vi "Text control 2 v3.2.vi"() -> ()   [LabVIEW 2016]
panel:
  out "I vs Vd":cluster{"Y data in":dbl[], "X data in":dbl[]}[](graph)
  in  "Auto Reset":bool
  in  "Reset":bool
  out "Id min vs time":cluster{"Y data in":dbl[], "X data in":dbl[]}[](graph)
  in  "Time Offset":dbl caption="Set Start Time (s)"
  out "Total lines":i32
  out "Line running":i32
  in  "byte count":u32=64
  in  "Serial End Mode for Reads":u16(ring)=2 items=["None", "LastBit", "TermChar"]
  in  "Timeout (ms)":u32=10000
  in  "Enable Termination\nChar (T)":bool=TRUE
  in  "Termination char\n(0xA = '\\n' = LF)\n(0xD = '\\r' = CR)":u8=13 format="%.0x"
  in  "flow control":u16(ring) items=["None"=0, "XON/XOFF"=1, "RTS/CTS"=2, "DTR/DSR"=4]
  in  "stop bits":u16(ring)=10 items=["1.0"=10, "1.5"=15, "2.0"=20]
  in  "parity":u16(ring) items=["None", "Odd", "Even", "Mark", "Space"]
  in  "data bits":u16=8 min=5 max=8 step=1
  in  "VISA resource name":refnum<visa-resource-name>="COM6"
  in  "baud rate":u32=9600
  out "Serial port output":string
  out "error out":errorcluster
  in  "Units":u16(ring) items=["Seconds", "Minutes", "Hours"]
  out "Elapsed Time":dbl caption="Elapsed Time (s)"
  out "Id max vs time":cluster{"Y data in":dbl[], "X data in":dbl[]}[](graph)
  out "Ig":dbl format="%.2e"
  out "Id":dbl format="%.2e"
  out "Is":dbl format="%.2e"
  out "I vs Vg":cluster{"Y data in":dbl[], "X data in":dbl[]}[](graph)
  in  "Panel Controls 2":T1={"Emergency Stop"=refnum, "TransGraph Max"=1e-05, "Text/Graph (text=false)"=TRUE, "TransGraph Min"=1e-11} {"TransGraph Min" format="%.2e"; "TransGraph Max" format="%.2e"}
  out "Command running:":string="#output s 0 0 0 -0.008 0.008 0.002"
  in  "Standby":T2
  in  "Full Reset":bool
  in  "SMU4":cluster{"on/off":bool, "Voltage":dbl} {"Voltage" min=-100.0 max=100.0 format="%.2f"}
  in  "Source/Drain Range":u8(slide)=6 max=11 scale=0.0..11.0
  in  "Source/Drain\nRange mode":u16(ring) items=["Auto", "Limited", "Fixed"]
  in  "Gate Range":u8(slide)=6 max=11 scale=0.0..11.0
  in  "Gate Range\nmode":u16(ring) items=["Auto", "Limited", "Fixed"]
  in  "Gate":T3={"Gate Start"=0.0, "Gate Stop"=2.0, "Gate Step (linear only)"=1.0, "Gate Compliance"=0.0001, "Gate PComp"=0.0, "Range mode"=0, "Range"=6} {"Range" max=11 scale=0.0..11.0; "Range mode" items=["Auto", "Limited", "Fixed"]; "Gate PComp" format="%^.2e"; "Gate Compliance" format="%^.2e"; "Gate Step (linear only)" format="%^.4e"; "Gate Stop" format="%^.4e"; "Gate Start" format="%^.4e"}
  in  "Drain 2":T4={"Drain Start"=0.0, "Drain Stop"=2.0, "Drain Compliance"=0.0001, "Drain Step"=1.0, "Drain PComp"=0.0, "Range mode"=0, "Range"=6} {"Range" max=11 scale=0.0..11.0; "Range mode" items=["Auto", "Limited", "Fixed"]; "Drain PComp" format="%^.2e"; "Drain Step" format="%^.4e"; "Drain Compliance" format="%^.2e"; "Drain Stop" format="%^.4e"; "Drain Start" format="%^.4e"}
  in  "Timings 2":T5={"integration time"=0, "Short/Long integration time"=0.00064, "hold time (sec)"=0.0, "delay time (sec)"=0.0, "Step Time (0 disables)"=0.0, "sweep method"=0, "Pulse period"=0.005, "Base voltage"=0.0, "Pulse width"=0.0005} {"Pulse width" min=0.0005 max=0.1 step=0.0001 format="%.4f"; "Base voltage" format="%^.4e"; "Pulse period" min=0.005 max=1.0 step=0.0001 format="%.4f"; "sweep method" items=["Continuous", "Pulsed"]; "Step Time (0 disables)" format="%.2f"; "delay time (sec)" format="%.4f"; "hold time (sec)" format="%.4f"; "Short/Long integration time" format="%^.0e"; "integration time" scale=0.0..2.0}
  in  "Panel Controls":T6={"Emergency Stop"=refnum, "TransGraph Max"=1e-05, "Text/Graph (text=false)"=TRUE} {"TransGraph Max" format="%.2e"}
  in  "Interrupt run":bool
  in  "Drain: Compliance":dbl=0.001 format="%.8f"
  in  "Gate: Compliance":dbl=0.001 format="%.8f"
  out "Path":path=path "C:/users/rlp38/09Apr2009LTtesting/test2.txt"
  in  "hold time /s":dbl format="%.2f"
  in  "delay time /s":dbl format="%.2f"
  in  "integration time":u32(slide) max=2 step=1 scale=0.0..2.0
  in  "Integration time (short)":dbl=0.0019 min=8e-05 max=0.0019 step=8e-05 format="%^.0e"
  in  "Integration time (long)":dbl=0.32 min=0.04 max=2.0 step=0.02 format="%.2f"
  in  "Step delay /s":dbl format="%.2f"
  in  "Program":string="#pulsedstressV d 0.03 20 0 0.5 0.0827 5\n#\n#itime s\n#gaterangemode l\n#drainrangemode l\n#pulsed on 0.05 0 0.02\n#transfer d 1 -1 -0.1 -1 -1 0\n#wait-min 1\n#transfer d 1 -1 -0.1 -1 -1 0\n#output d 0 -1 -0.5 0 -1 -0.1\n#transfer d -10 40 1 5 40 35\n#transfer d -10 40 1 5 40 35\n#output d 0 40 20 0 40 1\n#\n#\n#sample 1 0.008 221 6 0.003\n#samplei 400e-6 200 6 0.002 0.1\n#vsu2pulse -10 4\n#\n#stressV 0.016 0.03 2e-4 0.1e-3 11\n#stressI 220e-7 0.08 15\n#transfer s -1 1 0.5 -0.005 0.005 0.005\n#output s 0 0 0 -0.008 0.008 0.002\n"
  # "Serial port settings"
  # "Time"
  # "100 samples is approx 13s with medium integration"
  # "Syntax:\nitime [s|m|l]\ngaterangemode [a|l|f]\ndrainrangemode [a|l|f]\npulsed [on|off] PulsePeriod(sec) PulseBaseVoltage PulseONWidth(sec)\nstandby [on l off]\nwait NumMilliseconds\nwait-min NumMinutes\n# texthere = comment\ntransfer [s|d] VgStart VgStop VgStep VdStart VdStop VdStep\noutput [s|d] VgStart VgStop VgStep VdStart VdStop VdStep\nsample Vg Vd NumSamples Time(s) SampleInterval(s)\nsamplei Idg NumSamples Time(s) SampleInterval(s) VDGcompliance\n# if in doubt use SampleInterval(s) = 0.004\nstressV VG VD IGcompliance IDcompliance Duration(sec)\nstressI IDG VDGcompliance Duration(sec)\nvsu2pulse Bias Duration(s)\npulsedstressV [s|d] VEstop VgON VgOFF Period(s) PulseONwidth(s) Vd\nsample-fpp Vg Vd NumSamples Time\nresample-fpp Vg Vd\ntransfer-fpp [s|d] VgStart VgStop VgStep VdStart VdStop VdStep\noutput-fpp [s|d] VgStart VgStop VgStep VdStart VdStop VdStep\nserial SerialPortCommand"
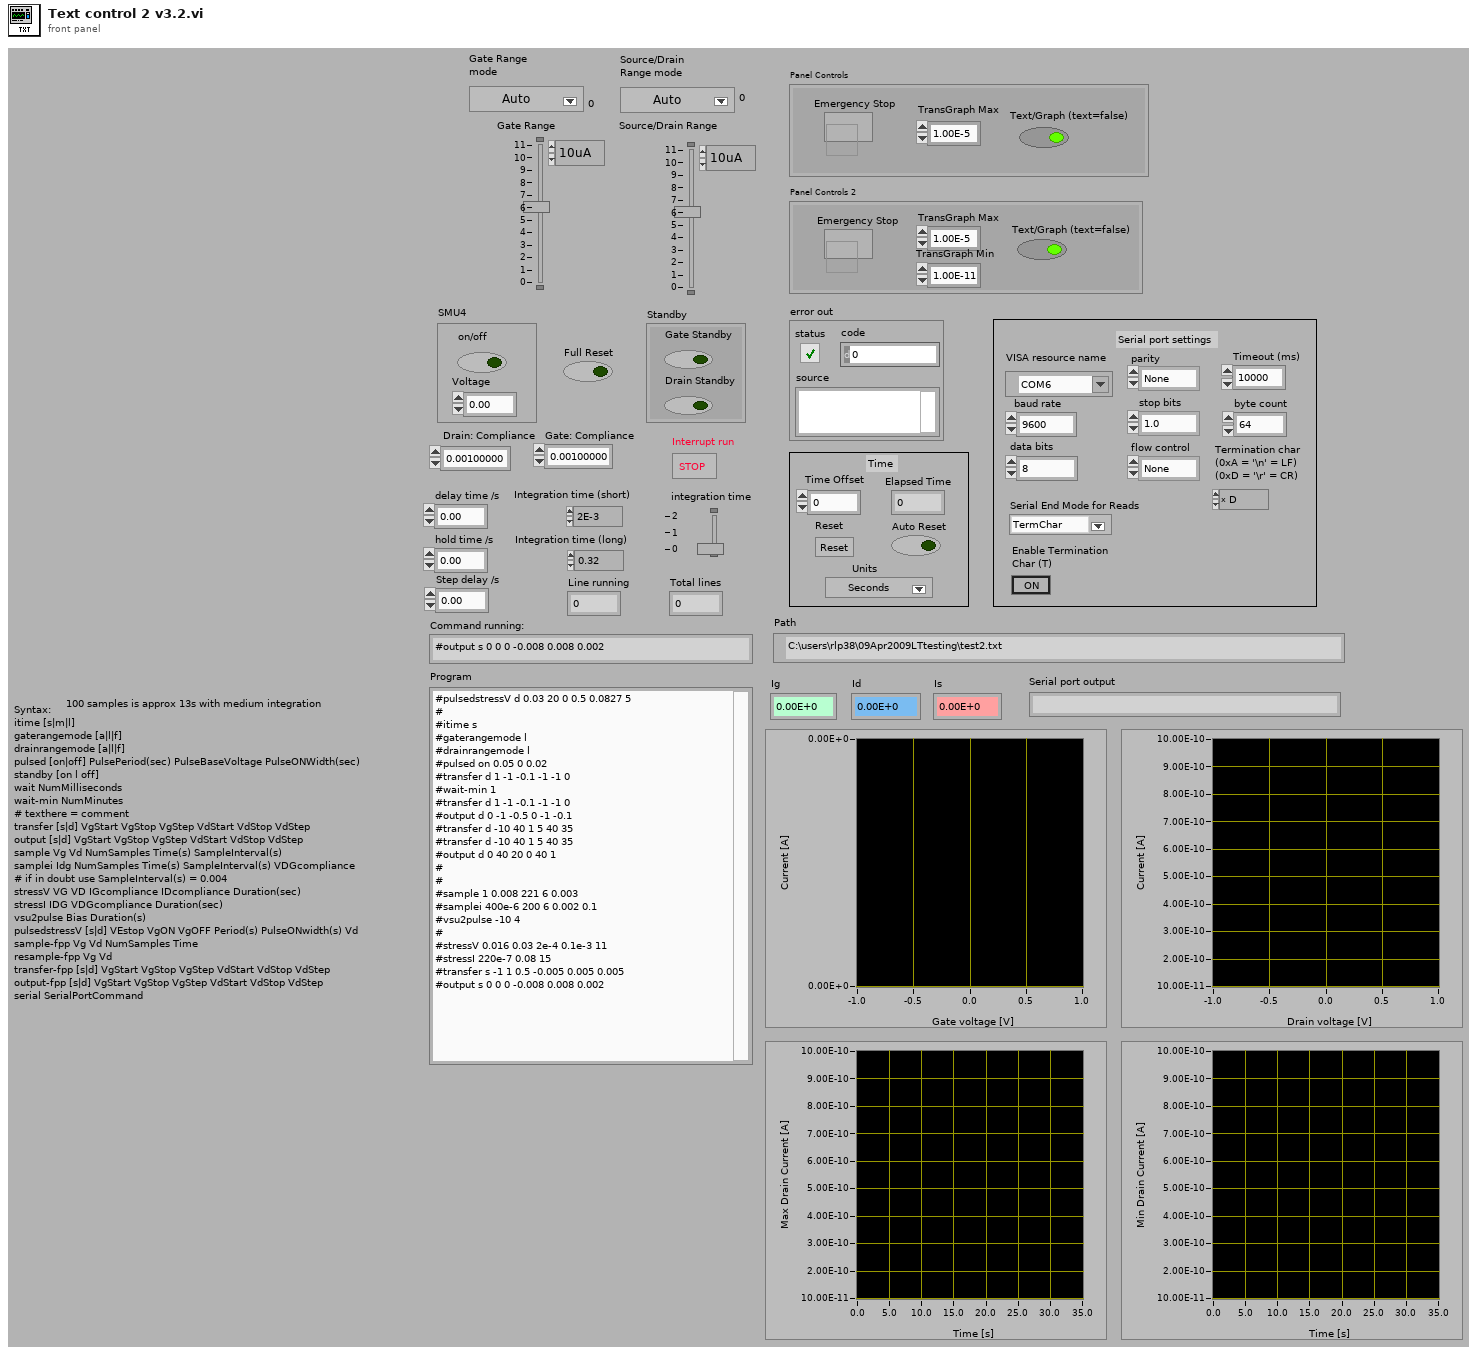
[diagram p1: front panel]
types:
  T1 = cluster{"Emergency Stop":refnum<vi>, "TransGraph Max":dbl, "Text/Graph (text=false)":bool, "TransGraph Min":dbl}
  T2 = cluster{"Gate Standby":bool, "Drain Standby":bool}
  T3 = cluster{"Gate Start":dbl, "Gate Stop":dbl, "Gate Step (linear only)":dbl, "Gate Compliance":dbl, "Gate PComp":dbl, "Range mode":u16, "Range":u8}
  T4 = cluster{"Drain Start":dbl, "Drain Stop":dbl, "Drain Compliance":dbl, "Drain Step":dbl, "Drain PComp":dbl, "Range mode":u16, "Range":u8}
  T5 = cluster{"integration time":u32, "Short/Long integration time":dbl, "hold time (sec)":dbl, "delay time (sec)":dbl, "Step Time (0 disables)":dbl, "sweep method":u16, "Pulse period":dbl, "Base voltage":dbl, "Pulse width":dbl}
  T6 = cluster{"Emergency Stop":refnum<vi>, "TransGraph Max":dbl, "Text/Graph (text=false)":bool}
  T7 = enum16{"open", "replace", "create", "open or create", "replace or create", "replace or create with confirmation"}
  T8 = cluster{"V2 Start":dbl, "V2 Step":dbl, "Number of points":i32}
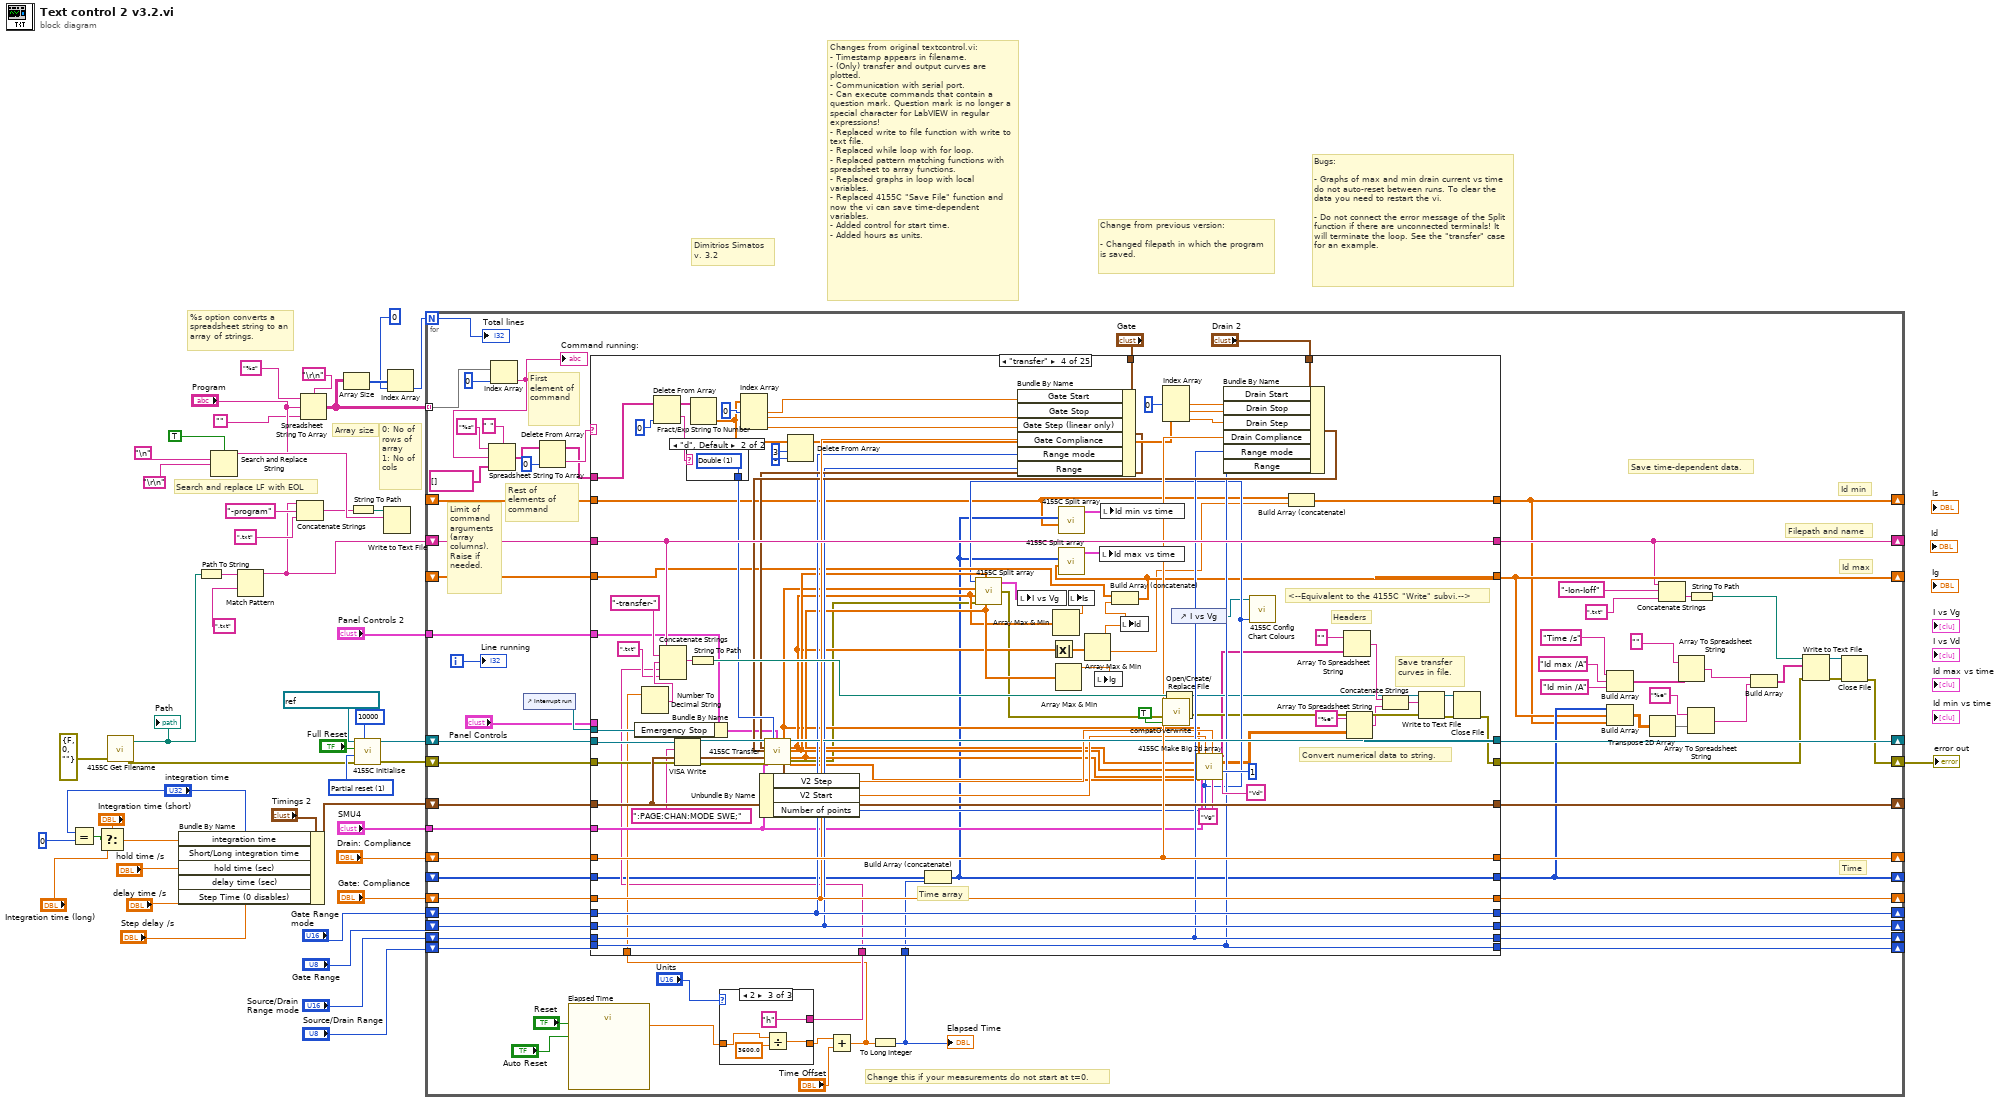
[diagram p0: block diagram]
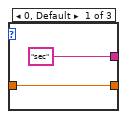
[diagram p2: hidden frame]
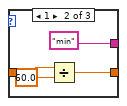
[diagram p3: hidden frame]
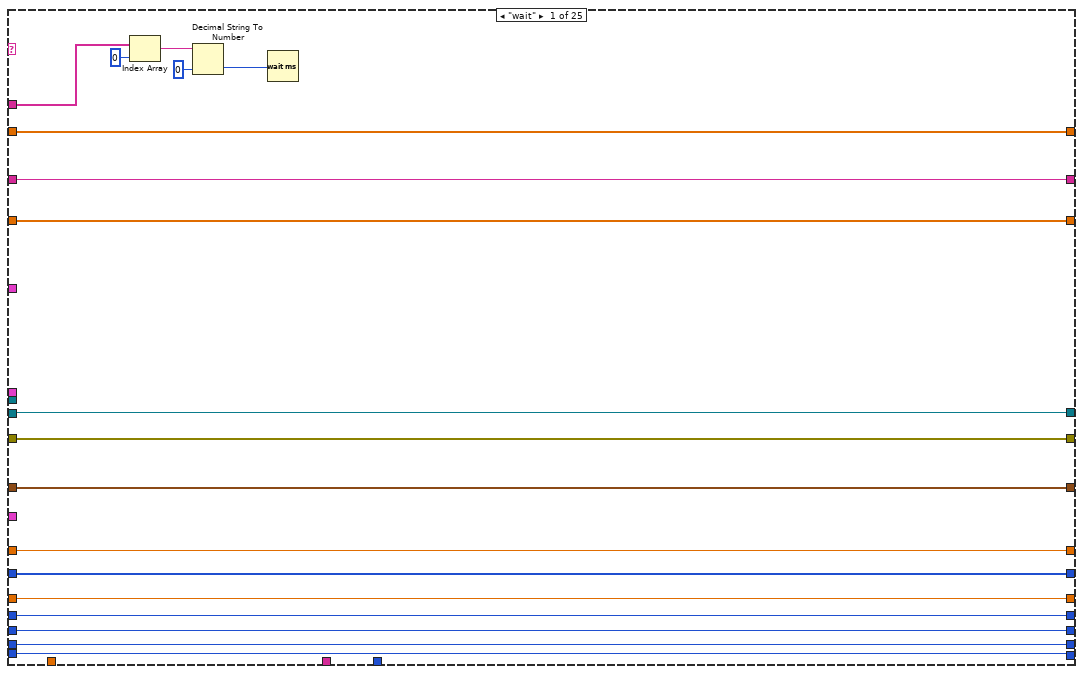
[diagram p4: hidden frame]
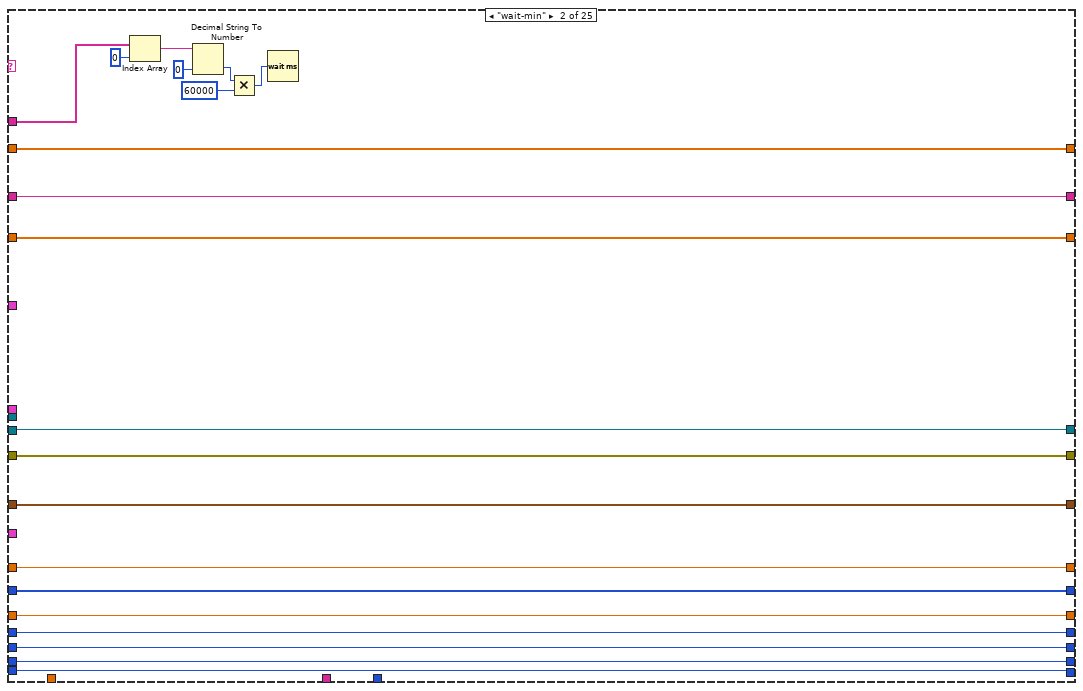
[diagram p5: hidden frame]
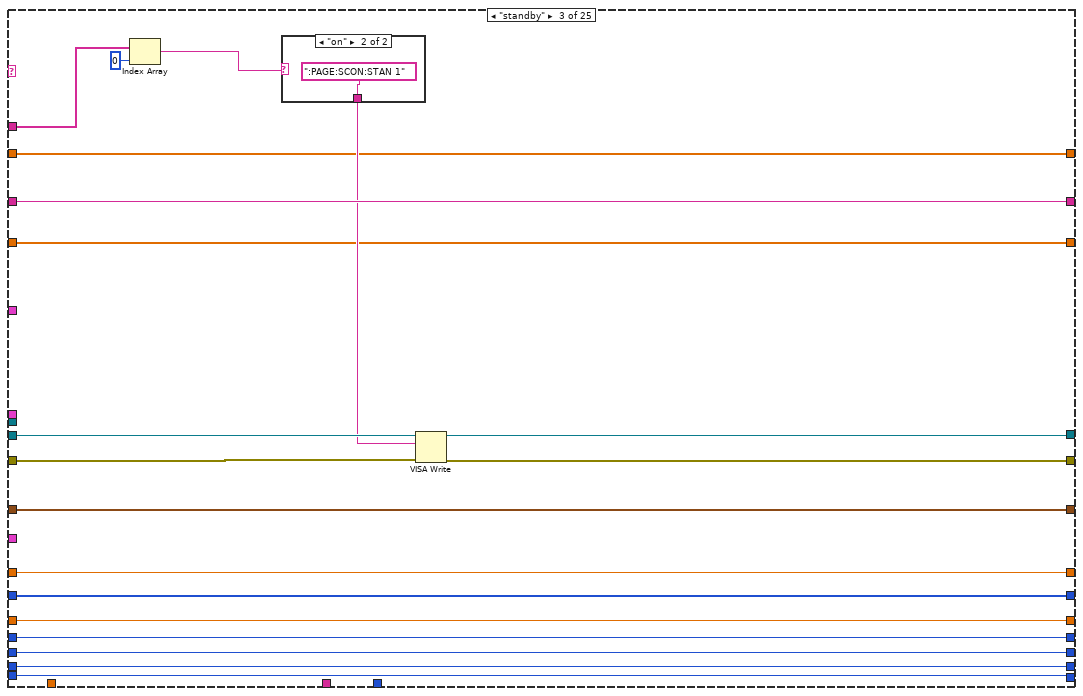
[diagram p6: hidden frame]
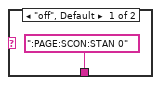
[diagram p7: hidden frame]
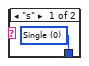
[diagram p8: hidden frame]
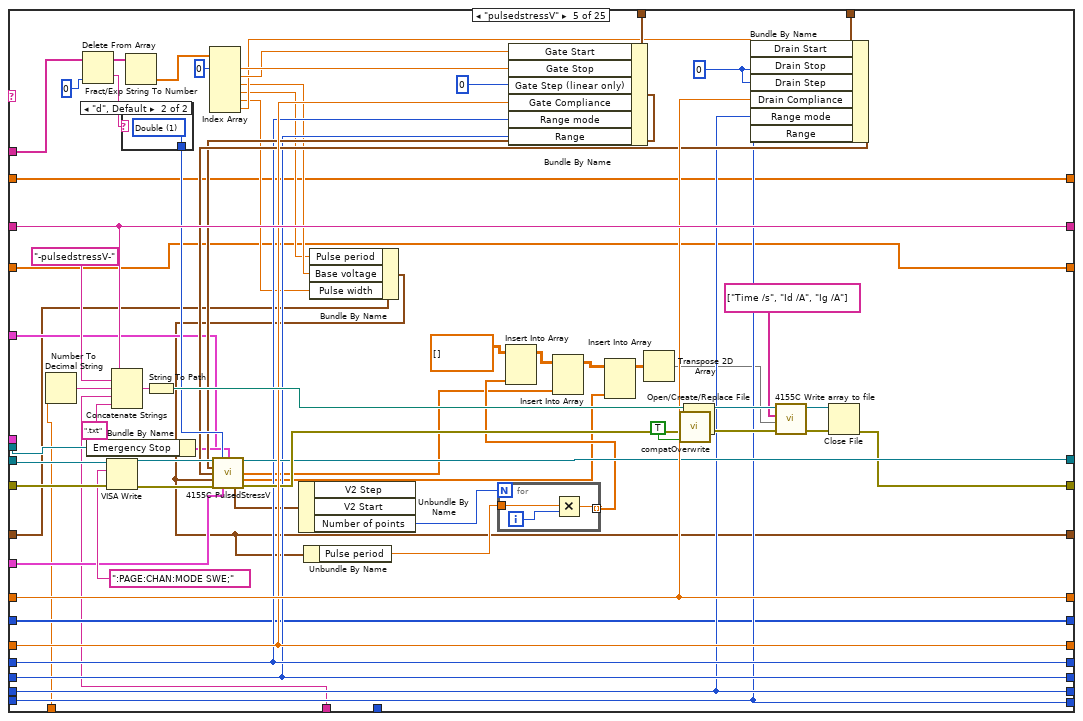
[diagram p9: hidden frame]
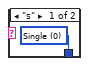
[diagram p10: hidden frame]
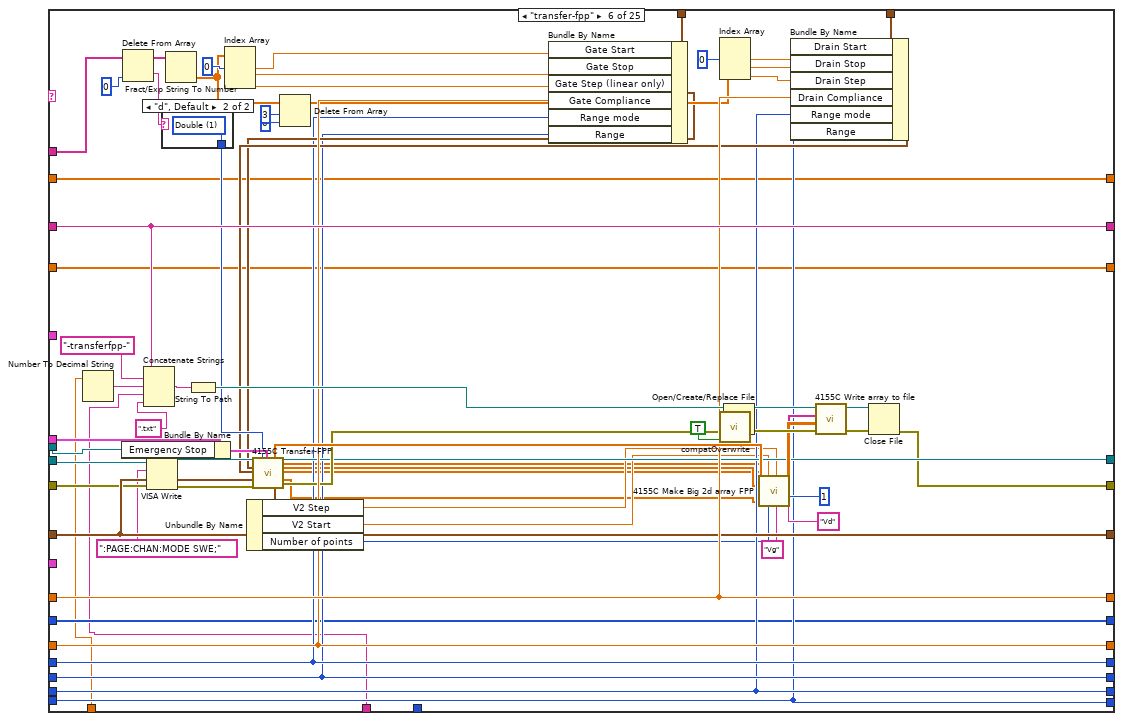
[diagram p11: hidden frame]
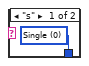
[diagram p12: hidden frame]
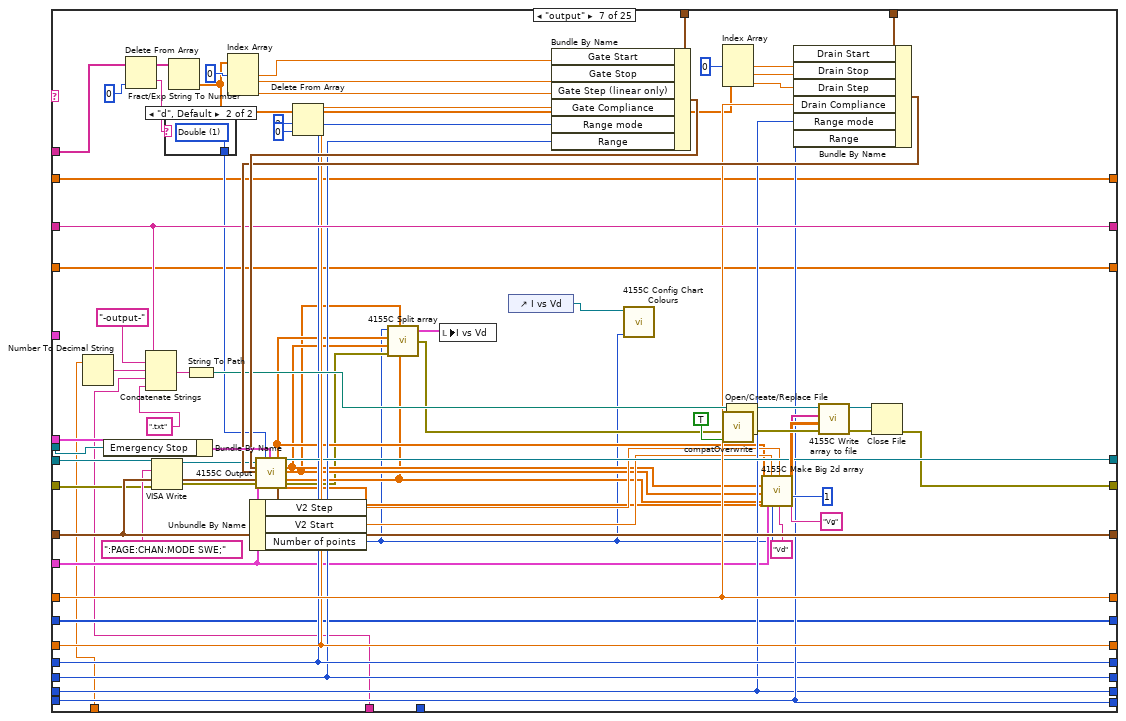
[diagram p13: hidden frame]
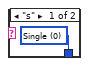
[diagram p14: hidden frame]
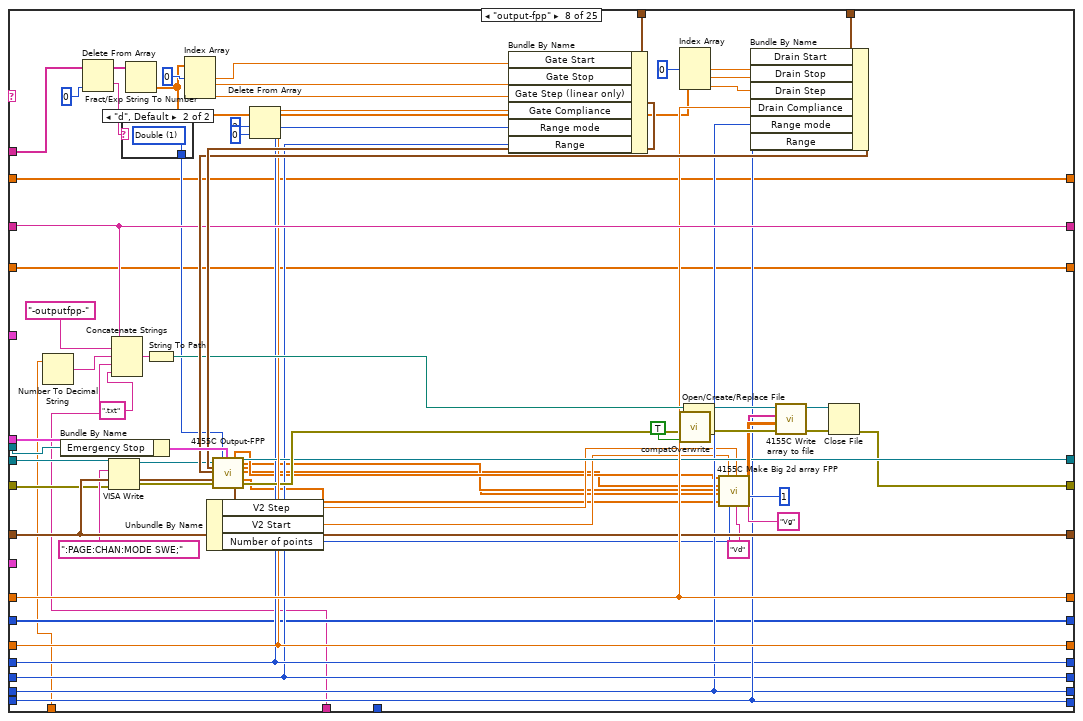
[diagram p15: hidden frame]
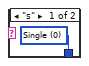
[diagram p16: hidden frame]
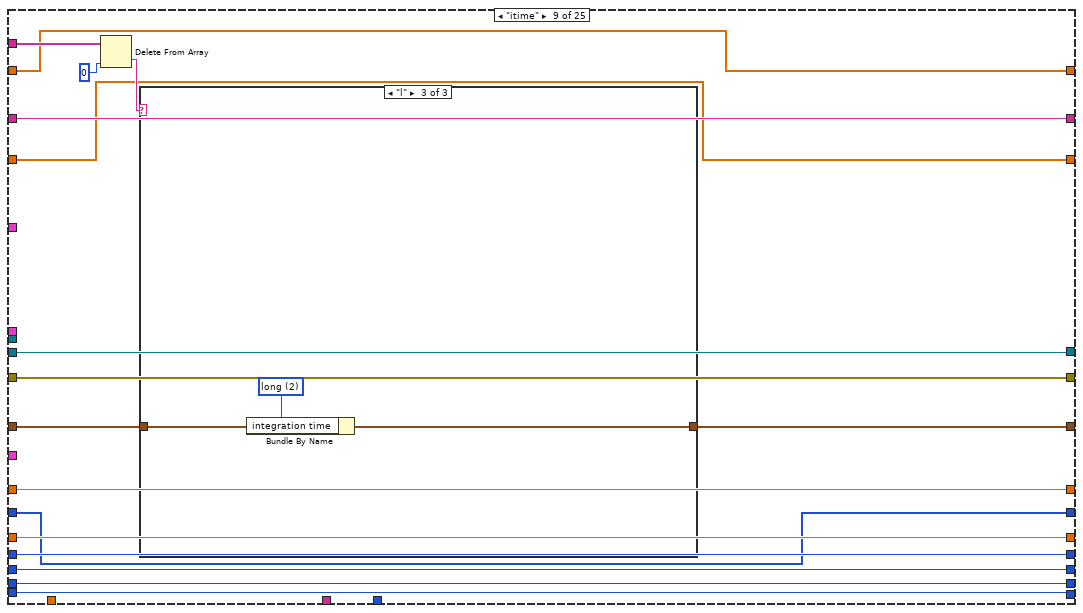
[diagram p17: hidden frame]
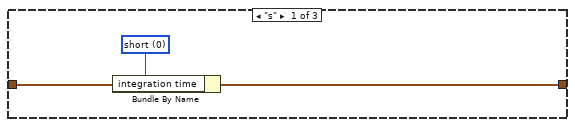
[diagram p18: hidden frame]
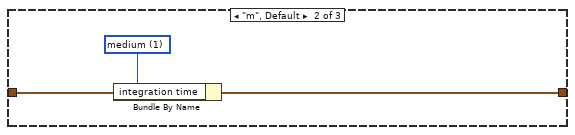
[diagram p19: hidden frame]
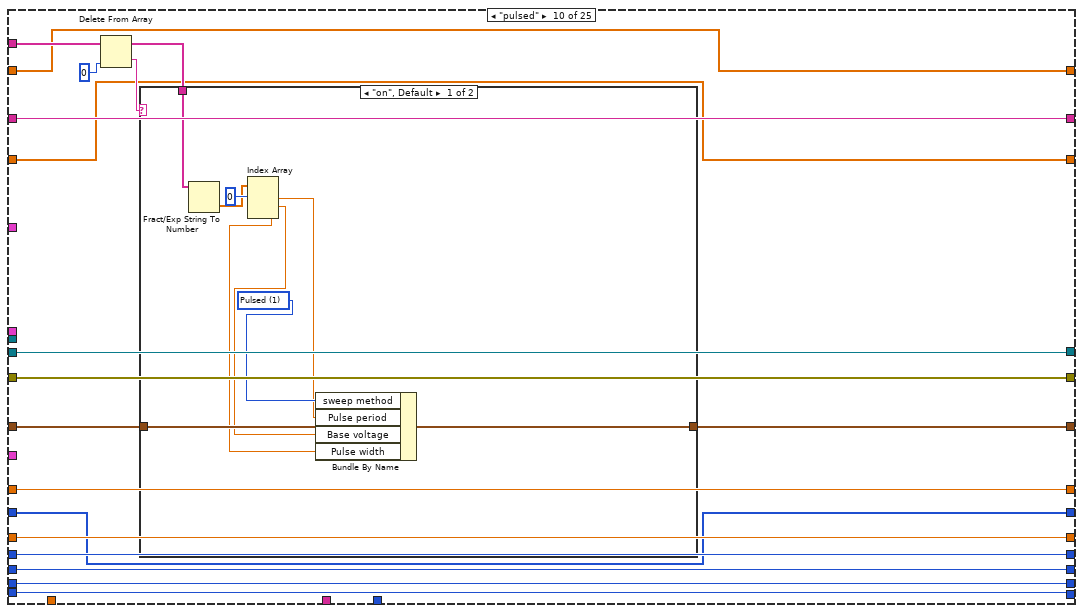
[diagram p20: hidden frame]
diagram:
  w39 = u16 1 items=["Reset All", "Partial reset"] ("Type of reset")
  # "Bugs:\n\n- Graphs of max and min drain current vs time do not auto-reset between runs. To clear the data you need to restart the vi.\n\n- Do not connect the error message of the Split function if there are unconnected terminals! It will terminate the loop. See the \"transfer\" case for an example."
  # "Array size"
  # "%s option converts a spreadsheet string to an array of strings."
  # "0: No of rows of array\n1: No of cols"
  # "Change from previous version:\n\n- Changed filepath in which the program is saved."
  # "Dimitrios Simatos\nv. 3.2"
  # "Changes from original textcontrol.vi:\n- Timestamp appears in filename.\n- (Only) transfer and output curves are plotted.\n- Communication with serial port.\n- Can execute commands that contain a question mark. Question mark is no longer a special character for LabVIEW in regular expressions!\n- Replaced write to file function with write to text file.\n- Replaced while loop with for loop.\n- Replaced pattern matching functions with spreadsheet to array functions.\n- Replaced graphs in loop with local variables.\n- Replaced 4155C \"Save File\" function and now the vi can save time-dependent variables.\n- Added control for start time.\n- Added hours as units."
  # "Search and replace LF with EOL"
  n1 = Equal?(x="integration time", y=u32 0) -> (x = y?=w43:bool)
  n2 = Select(t="Integration time (short)", s=w43, f="Integration time (long)") -> (s? t:f=w47:dbl)
  n3 = call "4155C Get Filename.vi"("error in (no error)"=errorcluster {"status"=FALSE, "code"=0, "source"=""}) -> ("error out"=w34:errorcluster, "path"=w8:path)  [unwired: 2 in, 1 out]
  "Path" <- w8
  n4 = Bundle By Name(cluster="Timings 2", "integration time"="integration time", "Short/Long integration time"=w47, "hold time (sec)"="hold time /s", "delay time (sec)"="delay time /s", "Step Time (0 disables)"="Step delay /s") -> (w31:T5)
  n5 = Path To String(path=w8) -> (string=w9:string)
  n6 = Search and Replace String(replace all?=TRUE ("replace all? (F)"), input string="Program", search string="\n", replace string="\r\n") -> (result string=w21:string)  [unwired: 4 in, 3 out]
  n7 = Match Pattern(string=w9, regular expression=".txt") -> (before substring=w3:string)  [unwired: 1 in, 3 out]
  n8 = Concatenate Strings(w3, "-program" ("Prefix"), ".txt" ("regular expression")) -> (w2:string)
  n9 = Spreadsheet String To Array(delimiter (Tab)="\r\n", format string="%s", spreadsheet string="Program", array type (2D Dbl)="") -> (array=w12:string[][])
  n10 = Array Size(array=w12) -> (size(s)=w16:i32[])
  n11 = String To Path(string=w2) -> (path=w1:path)
  n12 = call "4155C Initialise.vi"("VISA resource name in"=refnum<visa-resource-name> "GPIB0::14::INSTR", "Reset"="Full Reset", "Type of reset"=w39, "error in (no error)"=w34, "VISA Timeout Value"=u32 10000) -> ("VISA Resource Name out"=w33:refnum<visa-resource-name>, "error out"=w32:errorcluster)
  n13 = Write to Text File(file (use dialog)=w1, text=w21) -> ()  [unwired: 2 in, 3 out]
  n14 = Index Array(array=w16, index=0) -> (element=w14:i32)
  n15 = for {
    N: w14 -> [w86]
    tunnel: "SMU4" -> [w97]
    shift-left: "Source/Drain Range" -> [w102]
    shift-right: [w98] -> _
    shift-left: "Source/Drain\nRange mode" -> [w103]
    shift-right: [w99] -> _
    shift-left: "Gate Range" -> [w104]
    shift-right: [w100] -> _
    shift-left: "Gate Range\nmode" -> [w105]
    shift-right: [w101] -> _
    shift-left: "Gate: Compliance" -> [w114]
    shift-right: [w110] -> _
    shift-left: "Drain: Compliance" -> [w115]
    shift-right: [w111] -> _
    shift-left: w31 -> [w116]
    shift-right: [w112] -> _
    shift-left: w32 -> [w117]
    shift-right: [w56] -> w7
    shift-left: w33 -> [w118]
    shift-right: [w113] -> _
    shift-left: w3 -> [w119]
    shift-right: [w59] -> _
    tunnel: "Panel Controls 2" -> [w96]
    shift-right: [w62] -> _
    shift-left: _ -> [w95]
    shift-right: [w63] -> _
    shift-left: _ -> [w91]
    tunnel: w12 -> [w89] mode=indexing
    shift-right: [w54] -> _
    shift-left: _ -> [w55]
    i -> [w87]
    # "Filepath and name"
    # "Save time-dependent data."
    # "Change this if your measurements do not start at t=0."
    # "Time"
    # "Rest of elements of command"
    # "Id min"
    # "Id max"
    # "Limit of command arguments (array columns). Raise if needed."
    # "First element of command"
    n16 = Index Array(array=w89, index=0 ("line index")) -> (element=w82:string)
    "Command running:" <- w82
    n17 = Spreadsheet String To Array(delimiter (Tab)=" ", format string="%s", spreadsheet string=w82, array type (2D Dbl)=string[] []) -> (array=w79:string[])
    n18 = control-ref of="Interrupt run"() -> (w109:refnum<vi>)
    n19 = Delete From Array(array=w79, index=0) -> (deleted portion=w80:string, array with subset deleted=w78:string[])  [unwired: 1 in]
    n20 = call "Elapsed Time"("Reset"="Reset", "Auto Reset"="Auto Reset") -> ("Elapsed Time (s)"=w92:dbl)  [unwired: 10 in, 7 out]
    n21 = case shown="2" "Units" {
      tunnel: ["sec" "min" "h"] -> w93
      tunnel: [w120 w124 w127] -> w50
      tunnel: w92 -> [w120 w123 w128]
      frame 0, Default {
      }
      frame 1 {
        n22 = Divide(x=w123, y=60.0) -> (x/y=w124:dbl)
      }
      frame 2 {
        n23 = Divide(x=w128, y=3600.0) -> (x/y=w127:dbl)
      }
    }
    n24 = Add(x=w50, y="Time Offset") -> (x+y=w49:dbl)
    n25 = To Long Integer(number=w49) -> (32bit integer=w90:i32)
    "Elapsed Time" <- w90
    n26 = case shown="\"transfer\"" w80 {
      tunnel: w78 -> [w147 w167 w186 w267 w332 w402 w478 w549 w588 w615 w643 w669 w691 w706 _ _ w813 w875 _ w942 w987 w1030 w1101 w1164 w1172]
      tunnel: w119 -> [w142 w163 w184 w274 w339 w410 w485 w557 w577 w604 w635 w662 w685 w699 w719 w762 w791 w857 w889 w929 w974 w1018 w1095 w1160 w1174]
      tunnel: w118 -> [w141 w162 w175 w245 w323 w379 w454 w525 w578 w605 w636 w663 w686 w700 w724 w764 w819 w881 w893 w948 w993 w1036 w1107 w1118 w1178]
      tunnel: w117 -> [w140 w161 w174 w244 w322 w378 w451 w522 w579 w606 w637 w664 w687 w701 w723 w735 w818 w880 w892 w947 w992 w1035 w1106 w1117 w1177]
      tunnel: w116 -> [w139 w160 w183 w270 w298 w406 w481 w553 w587 w614 w634 w661 w684 w698 w722 w759 w782 w849 w898 w922 w967 w1011 w1094 w1159 w1179]
      tunnel: w115 -> [w138 w159 w182 w272 w337 w408 w483 w555 w586 w613 w642 w668 w690 w705 w721 w744 w817 w879 w901 w946 w991 w1034 w1105 w1168 w1180]
      tunnel: w114 -> [w137 w158 w181 w271 w336 w407 w482 w554 w585 w612 w641 w667 w689 w704 w720 w745 w792 w858 w900 w930 w975 w1019 w1096 w1161 w1182]
      tunnel: [w141 w162 w173 w269 w334 w404 w480 w551 w578 w605 w636 w663 w686 w700 w724 w764 w783 w831 w891 w923 w968 w1012 w1047 w1120 w1178] -> w113
      tunnel: [w140 w161 w172 w268 w333 w403 w479 w550 w579 w606 w637 w664 w687 w701 w723 w734 w793 w832 w890 w931 w976 w1020 w1046 w1119 w1176] -> w57
      tunnel: [w139 w160 w183 w270 w294 w406 w481 w553 w580 w607 w634 w661 w684 w698 w722 w759 w782 w849 w898 w922 w967 w1011 w1094 w1159 w1179] -> w112
      tunnel: [w138 w159 w182 w272 w337 w408 w483 w555 w586 w613 w642 w668 w690 w705 w721 w744 w817 w879 w901 w946 w991 w1034 w1105 w1168 w1180] -> w111
      tunnel: [w137 w158 w181 w271 w336 w407 w482 w554 w585 w612 w641 w667 w689 w704 w720 w745 w792 w858 w900 w930 w975 w1019 w1096 w1161 w1182] -> w110
      tunnel: [w142 w163 w184 w274 w339 w410 w485 w557 w577 w604 w635 w662 w685 w699 w719 w762 w791 w857 w889 w929 w974 w1018 w1095 w1160 w1174] -> w59
      tunnel: w109 -> [_ _ _ w277 w343 w415 w489 w561 _ _ _ _ _ _ _ _ w788 w854 _ w928 w973 w1017 w1067 w1136 _]
      tunnel: "Gate" -> [_ _ _ w254 w326 w389 w465 w536 _ _ _ _ _ _ _ _ _ _ _ _ _ _ _ _ _]
      tunnel: "Drain 2" -> [_ _ _ w253 w325 w388 w464 w535 _ _ _ _ _ _ _ _ _ _ _ _ _ _ _ _ _]
      tunnel: "Panel Controls" -> [_ _ _ _ _ w387 w463 w534 _ _ _ _ _ _ _ _ _ _ _ _ _ _ _ _ _]
      tunnel: w105 -> [w136 w157 w180 w238 w316 w372 w449 w520 w584 w611 _ w660 w683 w697 w718 w746 w778 w845 w894 w918 w963 w1007 w1090 w1155 w1183]
      tunnel: w104 -> [w135 w156 w179 w237 w315 w371 w448 w519 w583 w610 w640 _ w674 w703 w717 w747 w779 w846 w895 w919 w964 w1008 w1091 w1156 w1184]
      tunnel: w103 -> [w134 w155 w178 w236 w314 w370 w447 w518 w582 w609 w639 w666 w688 _ w716 w748 w780 w847 w896 w920 w965 w1009 w1092 w1157 w1185]
      tunnel: w102 -> [w133 w154 w177 w235 w313 w369 w450 w521 w581 w608 w638 w665 _ w702 w715 w749 w781 w848 w897 w921 w966 w1010 w1093 w1158 w1186]
      tunnel: [w136 w157 w180 w238 w316 w372 w449 w520 w584 w611 w633 w660 w683 w697 w718 w746 w778 w845 w894 w918 w963 w1007 w1090 w1155 w1183] -> w101
      tunnel: [w135 w156 w179 w237 w315 w371 w448 w519 w583 w610 w640 w652 w674 w703 w717 w747 w779 w846 w895 w919 w964 w1008 w1091 w1156 w1184] -> w100
      tunnel: [w134 w155 w178 w236 w314 w370 w447 w518 w582 w609 w639 w666 w688 w696 w716 w748 w780 w847 w896 w920 w965 w1009 w1092 w1157 w1185] -> w99
      tunnel: [w133 w154 w177 w235 w313 w369 w450 w521 w581 w608 w638 w665 w675 w702 w715 w749 w781 w848 w897 w921 w966 w1010 w1093 w1158 w1186] -> w98
      tunnel: w97 -> [_ _ _ w230 w310 _ w443 _ _ _ _ _ _ _ _ _ _ _ _ _ _ _ _ _ _]
      tunnel: w96 -> [_ _ _ w228 w309 _ _ _ _ _ _ _ _ _ _ _ _ _ _ _ _ _ _ _ _]
      tunnel: [w132 w150 w170 w196 w286 w359 w440 w507 w576 w602 w632 w651 w673 w695 w714 w730 w770 w829 w888 w907 w956 w1001 w1044 w1113 w1175] -> w62
      tunnel: w95 -> [w132 w150 w170 w219 w286 w359 w440 w507 w576 w602 w632 w651 w673 w695 w714 w730 w770 w829 w888 w907 w956 w1001 w1044 w1113 w1175]
      tunnel: w49 -> [_ _ _ w215 w283 w357 w437 w504 _ _ _ _ _ _ _ w728 w768 w826 _ w904 w953 w998 w1041 w1109 _]
      tunnel: w93 -> [_ _ _ w212 w282 w355 w436 w503 _ _ _ _ _ _ _ w726 w766 w825 _ w903 w952 w997 w1040 w1110 _]
      tunnel: w90 -> [_ _ _ w197 _ _ _ _ _ _ _ _ _ _ _ _ _ _ _ _ _ _ _ _ _]
      tunnel: [w131 w149 w169 w192 w285 w358 w439 w506 w575 w601 w631 w650 w672 w694 w713 w729 w769 w828 w887 w906 w955 w1000 w1043 w1112 w1181] -> w63
      tunnel: w91 -> [w131 w149 w169 w211 w285 w358 w439 w506 w575 w601 w631 w650 w672 w694 w713 w729 w769 w828 w887 w906 w955 w1000 w1043 w1112 w1181]
      tunnel: [w130 w148 w168 w190 w281 w354 w435 w502 w574 w600 w630 w649 w671 w693 w712 w725 w765 w824 w886 w902 w951 w996 w1039 w1108 w1169] -> w54
      tunnel: w55 -> [w130 w148 w168 w189 w281 w354 w435 w502 w574 w600 w630 w649 w671 w693 w712 w725 w765 w824 w886 w902 w951 w996 w1039 w1108 w1169]
      frame "wait" {
        n27 = Index Array(array=w147, index=0 ("Index")) -> (element=w145:string)
        n28 = Decimal String To Number(string=w145, default (0L)=u32 0) -> (number=w144:u32)  [unwired: 1 in, 1 out]
        n29 = Wait (ms)(milliseconds to wait=w144) -> ()  [unwired: 1 out]
      }
      frame "wait-min" {
        n30 = Index Array(array=w167, index=0 ("Index")) -> (element=w165:string)
        n31 = Decimal String To Number(string=w165, default (0L)=u32 0) -> (number=w153:u32)  [unwired: 1 in, 1 out]
        n32 = Multiply(x=w153, y=u32 60000) -> (x*y=w152:u32)
        n33 = Wait (ms)(milliseconds to wait=w152) -> ()  [unwired: 1 out]
      }
      frame "standby" {
        n34 = Index Array(array=w186, index=0 ("Index")) -> (element=w176:string)
        n35 = case shown="\"on\"" w176 {
          tunnel: [":PAGE:SCON:STAN 0" ":PAGE:SCON:STAN 1"] -> w171
          frame "off", Default {
          }
          frame "on" {
          }
        }
        n36 = VISA Write(VISA resource name=w175, write buffer=w171, error in (no error)=w174) -> (VISA resource name out=w173:refnum<visa-resource-name>, error out=w172:errorcluster)  [unwired: 1 out]
      }
      frame "transfer" {
        # "<--Equivalent to the 4155C \"Write\" subvi.-->"
        # "Headers"
        # "Convert numerical data to string."
        # "Save transfer curves in file."
        # "Time array"
        n37 = Bundle By Name(cluster=w228, "Emergency Stop"=w277) -> (w229:T1)
        n38 = Number To Decimal String(number=w215) -> (decimal integer string=w214:string)  [unwired: 1 in]
        n39 = Delete From Array(array=w267, index=0 ("Index")) -> (deleted portion=w265:string, array with subset deleted=w264:string[])  [unwired: 1 in]
        n40 = Concatenate Strings(w274, "-transfer-" ("Prefix"), w214, w212, ".txt" ("Suffix")) -> (w276:string)
        n41 = VISA Write(VISA resource name=w245, write buffer=":PAGE:CHAN:MODE SWE;" ("write buffer (\"\")"), error in (no error)=w244) -> (VISA resource name out=w242:refnum<visa-resource-name>, error out=w243:errorcluster)  [unwired: 1 out]
        n42 = case shown="\"d\", Default" w265 {
          tunnel: [w279 w280] -> w263
          frame "s" {
            w279 = u16 0 items=["Single", "Double"] ("sweep mode")
          }
          frame "d", Default {
            w280 = u16 1 items=["Single", "Double"] ("sweep mode")
          }
        }
        n43 = String To Path(string=w276) -> (path=w273:path)
        n44 = Fract/Exp String To Number(string=w264) -> (number=w249:dbl[])  [unwired: 3 in, 1 out]
        n45 = Index Array(array=w249, index #1=0 ("Index")) -> (element #1=w262:dbl, element #2=w261:dbl, element #3=w260:dbl)  [unwired: 2 in]
        n46 = Delete From Array(array=w249, length=3 ("Length"), index=0 ("Index")) -> (array with subset deleted=w247:dbl[])  [unwired: 1 out]
        n47 = Build Array (concatenate)(w211, w197) -> (w192:i32[])
        n48 = Bundle By Name(cluster=w254, "Gate Start"=w262, "Gate Stop"=w261, "Gate Step (linear only)"=w260, "Gate Compliance"=w271, "Range mode"=w238, "Range"=w237) -> (w239:T3)
        n49 = call "4155C Split array.vi"("X data in"=w192, "Y1 data in"=w189) -> ("Array of clusters"=w193:cluster{"Y data in":dbl[], "X data in":dbl[]}[])  [unwired: 5 in, 1 out]
        n50 = local write "Id min vs time"(w193) -> ()
        n51 = Index Array(array=w247, index #1=0 ("Index")) -> (element #1=w257:dbl, element #2=w256:dbl, element #3=w255:dbl)  [unwired: 2 in]
        n52 = call <vilib>:"compatOverwrite.vi"("overwrite (F)"=TRUE) -> ("overwrite?"=w227:T7)
        n53 = control-ref of="I vs Vg"() -> (w216:refnum<vi>)
        n54 = Bundle By Name(cluster=w253, "Drain Start"=w257, "Drain Stop"=w256, "Drain Step"=w255, "Drain Compliance"=w272, "Range mode"=w236, "Range"=w235) -> (w240:T4)
        n55 = call "4155C Transfer.vi"("VISA resource name in"=w242, "Gate"=w239, "Drain"=w240, "Timings"=w270, "error in (no error)"=w243, "SMU4"=w230, "sweep mode"=w263, "Panel Controls"=w229) -> ("VG"=w220:dbl[], "Outparams"=w234:T8, "VISA Resource Name out"=w269:refnum<visa-resource-name>, "IS"=w221:dbl[], "ID"=w226:dbl[], "IG"=w222:dbl[], "error out"=w207:errorcluster, "SMU4"=w231:dbl[])  [unwired: 12 in]
        n56 = Unbundle By Name(w234) -> ("V2 Step"=w233:dbl, "V2 Start"=w232:dbl, "Number of points"=w217:i32)
        n57 = call "4155C Split array.vi"("Number of VAR2 steps"=w217, "Y2 data in"=w226, "X data in"=w220, "Y1 data in"=w221, "Y3 data in"=w222, "error in (no error)"=w207) -> ("Array of clusters"=w210:cluster{"Y data in":dbl[], "X data in":dbl[]}[], "error out"=w208:errorcluster)  [unwired: 1 in]
        n58 = local write "I vs Vg"(w210) -> ()
        n59 = Absolute Value(x=w221) -> (abs(x)=w225:dbl[])
        n60 = Array Max & Min(array=w221) -> (max value=w223:dbl)  [unwired: 3 out]
        n61 = Array Max & Min(array=w222) -> (max value=w224:dbl)  [unwired: 3 out]
        n62 = local write "Is"(w223) -> ()
        n63 = Array Max & Min(array=w225) -> (max value=w218:dbl, min value=w191:dbl)  [unwired: 2 out]
        n64 = local write "Ig"(w224) -> ()
        n65 = Build Array (concatenate)(w219, w218) -> (w196:dbl[])
        n66 = call "4155C Split array.vi"("X data in"=w192, "Y1 data in"=w196) -> ("Array of clusters"=w209:cluster{"Y data in":dbl[], "X data in":dbl[]}[])  [unwired: 5 in, 1 out]
        n67 = local write "Id max vs time"(w209) -> ()
        n68 = local write "Id"(w218) -> ()
        n69 = Open/Create/Replace File(file path (use dialog)=w273, error in=w208, operation (0:open)=w227) -> (refnum out=w195:refnum<file>, error out=w204:errorcluster)  [unwired: 3 in, 1 out]
        n70 = call "4155C Make Big 2d array.vi"("1D Var1"=w220, "1d IS"=w221, "1d ID"=w226, "1d IG"=w222, "1d SMU4"=w231, "SMU4"=w230, "VAR2 START"=w232, "Number of VAR2 steps"=w217, "VAR2 STEP"=w233, "VAR1 Name"="Vg", "Decimal places in header"=i8 1, "VAR2 Name"="Vd") -> ("Header array"=w194:string[], "Data array"=w201:dbl[][])  [unwired: 14 in]
        n71 = call "4155C Config Chart Colours.vi"("Numeric"=w217, "XY Graph 2"=w216) -> ()  [unwired: 6 in]
        n72 = Build Array (concatenate)(w189, w191) -> (w190:dbl[])
        n73 = Array To Spreadsheet String(array=w194, 3:"" ("format string")) -> (spreadsheet string=w200:string)  [unwired: 1 in]
        n74 = Array To Spreadsheet String(array=w201, 3:"%e" ("format string")) -> (spreadsheet string=w203:string)  [unwired: 1 in]
        n75 = Concatenate Strings(w200, w203) -> (w202:string)
        n76 = Write to Text File(file (use dialog)=w195, text=w202, error in=w204) -> (refnum out=w206:refnum<file>, error out=w205:errorcluster)  [unwired: 1 in, 1 out]
        n77 = Close File(refnum=w206, error in=w205) -> (error out=w268:errorcluster)  [unwired: 1 out]
      }
      frame "pulsedstressV" {
        w292 = 0
        n78 = Number To Decimal String(number=w283) -> (decimal integer string=w340:string)  [unwired: 1 in]
        n79 = Delete From Array(array=w332, index=0 ("Index")) -> (deleted portion=w330:string, array with subset deleted=w329:string[])  [unwired: 1 in]
        n80 = Bundle By Name(cluster=w309, "Emergency Stop"=w343) -> (w311:T1)
        n81 = VISA Write(VISA resource name=w323, write buffer=":PAGE:CHAN:MODE SWE;" ("write buffer (\"\")"), error in (no error)=w322) -> (VISA resource name out=w320:refnum<visa-resource-name>, error out=w321:errorcluster)  [unwired: 1 out]
        n82 = Concatenate Strings(w339, "-pulsedstressV-" ("Substring"), w340, w282, ".txt" ("Substring")) -> (w342:string)
        n83 = case shown="\"d\", Default" w330 {
          tunnel: [w352 w353] -> w328
          frame "s" {
            w352 = u16 0 items=["Single", "Double"] ("sweep mode")
          }
          frame "d", Default {
            w353 = u16 1 items=["Single", "Double"] ("sweep mode")
          }
        }
        n84 = Fract/Exp String To Number(string=w329) -> (number=w324:dbl[])  [unwired: 3 in, 1 out]
        n85 = String To Path(string=w342) -> (path=w338:path)
        n86 = Index Array(array=w324, index #1=0 ("Index")) -> (element #1=w301:dbl, element #2=w300:dbl, element #3=w297:dbl, element #4=w296:dbl, element #5=w295:dbl, element #6=w299:dbl)  [unwired: 5 in]
        n87 = Bundle By Name(cluster=w298, "Pulse period"=w296, "Base voltage"=w297, "Pulse width"=w295) -> (w294:T5)
        n88 = Unbundle By Name(w294) -> ("Pulse period"=w302:dbl)
        n89 = Bundle By Name(cluster=w326, "Gate Start"=w300, "Gate Stop"=w301, "Gate Step (linear only)"=0, "Gate Compliance"=w336, "Range mode"=w316, "Range"=w315) -> (w317:T3)
        n90 = call <vilib>:"compatOverwrite.vi"("overwrite (F)"=TRUE) -> ("overwrite?"=w287:T7)
        n91 = Bundle By Name(cluster=w325, "Drain Start"=w299, "Drain Stop"=w292, "Drain Step"=w292, "Drain Compliance"=w337, "Range mode"=w314, "Range"=w313) -> (w318:T4)
        n92 = call "4155C PulsedStressV.vi"("VISA resource name in"=w320, "sweep mode"=w328, "Panel Controls"=w311, "Gate"=w317, "Drain"=w318, "Timings"=w294, "error in (no error)"=w321, "SMU4"=w310) -> ("VISA Resource Name out"=w334:refnum<visa-resource-name>, "ID"=w290:dbl[], "IG"=w288:dbl[], "Outparams"=w312:T8, "error out"=w335:errorcluster)  [unwired: 3 in]
        n93 = Unbundle By Name(w312) -> ("Number of points"=w289:i32)  [unwired: 2 out]
        n94 = for {
          N: w289 -> [_]
          tunnel: [w349] -> w291 mode=indexing
          tunnel: w302 -> [w351]
          i -> [w350]
          n95 = Multiply(x=w351, y=w350) -> (x*y=w349:dbl)
        }
        n96 = Insert Into Array(array=dbl[][] [] ("Input Array"), new element=w291) -> (w303:dbl[][])  [unwired: 2 in]
        n97 = Insert Into Array(array=w303, new element=w290) -> (w308:dbl[][])  [unwired: 2 in]
        n98 = Insert Into Array(array=w308, new element=w288) -> (w307:dbl[][])  [unwired: 2 in]
        n99 = Transpose 2D Array(2D array=w307) -> (transposed array=w306:dbl[][])
        n100 = Open/Create/Replace File(file path (use dialog)=w338, error in=w335, operation (0:open)=w287) -> (refnum out=w346:refnum<file>, error out=w347:errorcluster)  [unwired: 3 in, 1 out]
        n101 = call "4155C Write array to file.vi"("Byte Stream File Refnum"=w346, "Header"=string[] ["Time /s", "Id /A", "Ig /A"], "Data Array"=w306, "error in (no error)"=w347) -> ("dup refnum"=w344:refnum<file>, "error out"=w345:errorcluster)  [unwired: 1 in]
        n102 = Close File(refnum=w344, error in=w345) -> (error out=w333:errorcluster)  [unwired: 1 out]
      }
      frame "transfer-fpp" {
        n103 = Number To Decimal String(number=w357) -> (decimal integer string=w411:string)  [unwired: 1 in]
        n104 = Bundle By Name(cluster=w387, "Emergency Stop"=w415) -> (w423:T6)
        n105 = Delete From Array(array=w402, index=0 ("Index")) -> (deleted portion=w400:string, array with subset deleted=w399:string[])  [unwired: 1 in]
        n106 = Concatenate Strings(w410, "-transferfpp-" ("Substring"), w411, w355, ".txt" ("Substring")) -> (w413:string)
        n107 = VISA Write(VISA resource name=w379, write buffer=":PAGE:CHAN:MODE SWE;" ("write buffer (\"\")"), error in (no error)=w378) -> (VISA resource name out=w376:refnum<visa-resource-name>, error out=w377:errorcluster)  [unwired: 1 out]
        n108 = case shown="\"d\", Default" w400 {
          tunnel: [w424 w425] -> w398
          frame "s" {
            w424 = u16 0 items=["Single", "Double"] ("sweep mode")
          }
          frame "d", Default {
            w425 = u16 1 items=["Single", "Double"] ("sweep mode")
          }
        }
        n109 = Fract/Exp String To Number(string=w399) -> (number=w383:dbl[])  [unwired: 3 in, 1 out]
        n110 = String To Path(string=w413) -> (path=w409:path)
        n111 = Index Array(array=w383, index #1=0 ("Index")) -> (element #1=w397:dbl, element #2=w396:dbl, element #3=w395:dbl)  [unwired: 2 in]
        n112 = Delete From Array(array=w383, length=3 ("Length"), index=0 ("Index")) -> (array with subset deleted=w381:dbl[])  [unwired: 1 out]
        n113 = Bundle By Name(cluster=w389, "Gate Start"=w397, "Gate Stop"=w396, "Gate Step (linear only)"=w395, "Gate Compliance"=w407, "Range mode"=w372, "Range"=w371) -> (w373:T3)
        n114 = Index Array(array=w381, index #1=0 ("Index")) -> (element #1=w392:dbl, element #2=w391:dbl, element #3=w390:dbl)  [unwired: 2 in]
        n115 = call <vilib>:"compatOverwrite.vi"("overwrite (F)"=TRUE) -> ("overwrite?"=w360:T7)
        n116 = Bundle By Name(cluster=w388, "Drain Start"=w392, "Drain Stop"=w391, "Drain Step"=w390, "Drain Compliance"=w408, "Range mode"=w370, "Range"=w369) -> (w374:T4)
        n117 = call "4155C Transfer-FPP.vi"("VISA resource name in"=w376, "Gate"=w373, "Drain"=w374, "Timings"=w406, "error in (no error)"=w377, "sweep mode"=w398, "Panel Controls"=w423) -> ("VG"=w414:dbl[], "Outparams"=w368:T8, "VISA Resource Name out"=w404:refnum<visa-resource-name>, "Vprobe2"=w364:dbl[], "ID"=w363:dbl[], "IG"=w362:dbl[], "Vprobe1"=w361:dbl[], "error out"=w405:errorcluster)  [unwired: 13 in]
        n118 = Unbundle By Name(w368) -> ("V2 Step"=w367:dbl, "V2 Start"=w366:dbl, "Number of points"=w365:i32)
        n119 = Open/Create/Replace File(file path (use dialog)=w409, error in=w405, operation (0:open)=w360) -> (refnum out=w420:refnum<file>, error out=w421:errorcluster)  [unwired: 3 in, 1 out]
        n120 = call "4155C Make Big 2d array FPP.vi"("1D Var1"=w414, "1d ID"=w363, "1d Vp2"=w364, "1d IG"=w362, "1d Vp1"=w361, "VAR2 START"=w366, "Number of VAR2 steps"=w365, "VAR2 STEP"=w367, "VAR1 Name"="Vg", "Decimal places in header"=i8 1, "VAR2 Name"="Vd") -> ("Header array"=w416:string[], "Data array"=w417:dbl[][])  [unwired: 15 in]
        n121 = call "4155C Write array to file.vi"("Byte Stream File Refnum"=w420, "Header"=w416, "Data Array"=w417, "error in (no error)"=w421) -> ("dup refnum"=w418:refnum<file>, "error out"=w419:errorcluster)  [unwired: 1 in]
        n122 = Close File(refnum=w418, error in=w419) -> (error out=w403:errorcluster)  [unwired: 1 out]
      }
      frame "output" {
        n123 = Number To Decimal String(number=w437) -> (decimal integer string=w486:string)  [unwired: 1 in]
        n124 = Bundle By Name(cluster=w463, "Emergency Stop"=w489) -> (w499:T6)
        n125 = Delete From Array(array=w478, index=0 ("Index")) -> (deleted portion=w476:string, array with subset deleted=w475:string[])  [unwired: 1 in]
        n126 = Concatenate Strings(w485, "-output-" ("Substring"), w486, w436, ".txt" ("Substring")) -> (w488:string)
        n127 = VISA Write(VISA resource name=w454, write buffer=":PAGE:CHAN:MODE SWE;" ("write buffer (\"\")"), error in (no error)=w451) -> (VISA resource name out=w453:refnum<visa-resource-name>, error out=w452:errorcluster)  [unwired: 1 out]
        n128 = case shown="\"d\", Default" w476 {
          tunnel: [w500 w501] -> w474
          frame "s" {
            w500 = u16 0 items=["Single", "Double"] ("sweep mode")
          }
          frame "d", Default {
            w501 = u16 1 items=["Single", "Double"] ("sweep mode")
          }
        }
        n129 = Fract/Exp String To Number(string=w475) -> (number=w457:dbl[])  [unwired: 3 in, 1 out]
        n130 = String To Path(string=w488) -> (path=w484:path)
        n131 = Index Array(array=w457, index #1=0 ("Index")) -> (element #1=w473:dbl, element #2=w472:dbl, element #3=w471:dbl)  [unwired: 2 in]
        n132 = Delete From Array(array=w457, length=3 ("Length"), index=0 ("Index")) -> (array with subset deleted=w456:dbl[])  [unwired: 1 out]
        n133 = control-ref of="I vs Vd"() -> (w427:refnum<vi>)
        n134 = Bundle By Name(cluster=w465, "Gate Start"=w473, "Gate Stop"=w472, "Gate Step (linear only)"=w471, "Gate Compliance"=w482, "Range mode"=w449, "Range"=w448) -> (w498:T3)
        n135 = Index Array(array=w456, index #1=0 ("Index")) -> (element #1=w468:dbl, element #2=w467:dbl, element #3=w466:dbl)  [unwired: 2 in]
        n136 = call <vilib>:"compatOverwrite.vi"("overwrite (F)"=TRUE) -> ("overwrite?"=w441:T7)
        n137 = Bundle By Name(cluster=w464, "Drain Start"=w468, "Drain Stop"=w467, "Drain Step"=w466, "Drain Compliance"=w483, "Range mode"=w447, "Range"=w450) -> (w497:T4)
        n138 = call "4155C Output.vi"("VISA resource name in"=w453, "Gate"=w498, "Drain"=w497, "Timings"=w481, "error in (no error)"=w452, "SMU4"=w443, "sweep mode"=w474, "Panel controls"=w499) -> ("VD"=w434:dbl[], "Outparams"=w445:T8, "VISA Resource Name out"=w480:refnum<visa-resource-name>, "IS"=w433:dbl[], "ID"=w432:dbl[], "IG"=w431:dbl[], "error out"=w429:errorcluster, "SMU4"=w442:dbl[])  [unwired: 12 in]
        n139 = Unbundle By Name(w445) -> ("V2 Step"=w446:dbl, "V2 Start"=w444:dbl, "Number of points"=w426:i32)
        n140 = call "4155C Split array.vi"("Number of VAR2 steps"=w426, "Y2 data in"=w432, "X data in"=w434, "Y1 data in"=w433, "Y3 data in"=w431, "error in (no error)"=w429) -> ("Array of clusters"=w430:cluster{"Y data in":dbl[], "X data in":dbl[]}[], "error out"=w428:errorcluster)  [unwired: 1 in]
        n141 = local write "I vs Vd"(w430) -> ()
        n142 = call "4155C Config Chart Colours.vi"("Numeric"=w426, "XY Graph 2"=w427) -> ()  [unwired: 6 in]
        n143 = Open/Create/Replace File(file path (use dialog)=w484, error in=w428, operation (0:open)=w441) -> (refnum out=w494:refnum<file>, error out=w495:errorcluster)  [unwired: 3 in, 1 out]
        n144 = call "4155C Make Big 2d array.vi"("1D Var1"=w434, "1d IS"=w433, "1d ID"=w432, "1d IG"=w431, "1d SMU4"=w442, "SMU4"=w443, "VAR2 START"=w444, "Number of VAR2 steps"=w426, "VAR2 STEP"=w446, "VAR1 Name"="Vd", "Decimal places in header"=i8 1, "VAR2 Name"="Vg") -> ("Header array"=w490:string[], "Data array"=w491:dbl[][])  [unwired: 14 in]
        n145 = call "4155C Write array to file.vi"("Byte Stream File Refnum"=w494, "Header"=w490, "Data Array"=w491, "error in (no error)"=w495) -> ("dup refnum"=w492:refnum<file>, "error out"=w493:errorcluster)  [unwired: 1 in]
        n146 = Close File(refnum=w492, error in=w493) -> (error out=w479:errorcluster)  [unwired: 1 out]
      }
      frame "output-fpp" {
        n147 = Number To Decimal String(number=w504) -> (decimal integer string=w558:string)  [unwired: 1 in]
        n148 = Bundle By Name(cluster=w534, "Emergency Stop"=w561) -> (w571:T6)
        n149 = Delete From Array(array=w549, index=0 ("Index")) -> (deleted portion=w547:string, array with subset deleted=w546:string[])  [unwired: 1 in]
        n150 = VISA Write(VISA resource name=w525, write buffer=":PAGE:CHAN:MODE SWE;" ("write buffer (\"\")"), error in (no error)=w522) -> (VISA resource name out=w524:refnum<visa-resource-name>, error out=w523:errorcluster)  [unwired: 1 out]
        n151 = Concatenate Strings(w557, "-outputfpp-" ("Substring"), w558, w503, ".txt" ("Substring")) -> (w560:string)
        n152 = case shown="\"d\", Default" w547 {
          tunnel: [w572 w573] -> w545
          frame "s" {
            w572 = u16 0 items=["Single", "Double"] ("sweep mode")
          }
          frame "d", Default {
            w573 = u16 1 items=["Single", "Double"] ("sweep mode")
          }
        }
        n153 = Fract/Exp String To Number(string=w546) -> (number=w528:dbl[])  [unwired: 3 in, 1 out]
        n154 = String To Path(string=w560) -> (path=w556:path)
        n155 = Index Array(array=w528, index #1=0 ("Index")) -> (element #1=w544:dbl, element #2=w543:dbl, element #3=w542:dbl)  [unwired: 2 in]
        n156 = Delete From Array(array=w528, length=3 ("Length"), index=0 ("Index")) -> (array with subset deleted=w527:dbl[])  [unwired: 1 out]
        n157 = Bundle By Name(cluster=w536, "Gate Start"=w544, "Gate Stop"=w543, "Gate Step (linear only)"=w542, "Gate Compliance"=w554, "Range mode"=w520, "Range"=w519) -> (w570:T3)
        n158 = Index Array(array=w527, index #1=0 ("Index")) -> (element #1=w539:dbl, element #2=w538:dbl, element #3=w537:dbl)  [unwired: 2 in]
        n159 = call <vilib>:"compatOverwrite.vi"("overwrite (F)"=TRUE) -> ("overwrite?"=w508:T7)
        n160 = Bundle By Name(cluster=w535, "Drain Start"=w539, "Drain Stop"=w538, "Drain Step"=w537, "Drain Compliance"=w555, "Range mode"=w518, "Range"=w521) -> (w569:T4)
        n161 = call "4155C Output-FPP.vi"("VISA resource name in"=w524, "Gate"=w570, "Drain"=w569, "Timings"=w553, "error in (no error)"=w523, "sweep mode"=w545, "Panel controls"=w571) -> ("VD"=w513:dbl[], "Outparams"=w516:T8, "VISA Resource Name out"=w551:refnum<visa-resource-name>, "Vprobe2"=w512:dbl[], "ID"=w511:dbl[], "IG"=w510:dbl[], "Vprobe1"=w509:dbl[], "error out"=w552:errorcluster)  [unwired: 13 in]
        n162 = Unbundle By Name(w516) -> ("V2 Step"=w517:dbl, "V2 Start"=w515:dbl, "Number of points"=w514:i32)
        n163 = Open/Create/Replace File(file path (use dialog)=w556, error in=w552, operation (0:open)=w508) -> (refnum out=w566:refnum<file>, error out=w567:errorcluster)  [unwired: 3 in, 1 out]
        n164 = call "4155C Make Big 2d array FPP.vi"("1D Var1"=w513, "1d ID"=w511, "1d Vp2"=w512, "1d IG"=w510, "1d Vp1"=w509, "VAR2 START"=w515, "Number of VAR2 steps"=w514, "VAR2 STEP"=w517, "VAR1 Name"="Vd", "Decimal places in header"=i8 1, "VAR2 Name"="Vg") -> ("Header array"=w562:string[], "Data array"=w563:dbl[][])  [unwired: 15 in]
        n165 = call "4155C Write array to file.vi"("Byte Stream File Refnum"=w566, "Header"=w562, "Data Array"=w563, "error in (no error)"=w567) -> ("dup refnum"=w564:refnum<file>, "error out"=w565:errorcluster)  [unwired: 1 in]
        n166 = Close File(refnum=w564, error in=w565) -> (error out=w550:errorcluster)  [unwired: 1 out]
      }
      frame "itime" {
        n167 = Delete From Array(array=w588, index=0 ("Index")) -> (deleted portion=w589:string)  [unwired: 1 in, 1 out]
        n168 = case shown="\"l\"" w589 {
          tunnel: w587 -> [w593 w595 w598]
          tunnel: [w592 w594 w597] -> w580
          frame "s" {
            w591 = u32 0 items=["short  ", "medium  ", "long  "] ("integration time 2")
            n169 = Bundle By Name(cluster=w593, "integration time"=w591) -> (w592:T5)
          }
          frame "m", Default {
            w596 = u32 1 items=["short  ", "medium  ", "long  "] ("integration time 2")
            n170 = Bundle By Name(cluster=w595, "integration time"=w596) -> (w594:T5)
          }
          frame "l" {
            w599 = u32 2 items=["short  ", "medium  ", "long  "] ("integration time 2")
            n171 = Bundle By Name(cluster=w598, "integration time"=w599) -> (w597:T5)
          }
        }
      }
      frame "pulsed" {
        n172 = Delete From Array(array=w615, index=0 ("Index")) -> (deleted portion=w616:string, array with subset deleted=w603:string[])  [unwired: 1 in]
        n173 = case shown="\"on\", Default" w616 {
          tunnel: w614 -> [w626 w629]
          tunnel: [w625 w628] -> w607
          tunnel: w603 -> [w623 _]
          frame "on", Default {
            w624 = u16 1 items=["Continuous", "Pulsed"] ("sweep method")
            n174 = Fract/Exp String To Number(string=w623) -> (number=w621:dbl[])  [unwired: 3 in, 1 out]
            n175 = Index Array(array=w621, index #1=0 ("Index")) -> (element #1=w620:dbl, element #2=w619:dbl, element #3=w618:dbl)  [unwired: 2 in]
            n176 = Bundle By Name(cluster=w626, "sweep method"=w624, "Pulse period"=w620, "Base voltage"=w619, "Pulse width"=w618) -> (w625:T5)
          }
          frame "off" {
            w627 = u16 0 items=["Continuous", "Pulsed"] ("sweep method")
            n177 = Bundle By Name(cluster=w629, "sweep method"=w627) -> (w628:T5)
          }
        }
      }
      frame "gaterangemode" {
        n178 = Delete From Array(array=w643, index=0 ("Index")) -> (deleted portion=w644:string)  [unwired: 1 in, 1 out]
        n179 = case shown="\"f\"" w644 {
          tunnel: [w646 w647 w648] -> w633
          frame "a", Default {
            w646 = u16 0 items=["Auto", "Limited", "Fixed"] ("Gate Range\nmode 2")
          }
          frame "f" {
            w647 = u16 2 items=["Auto", "Limited", "Fixed"] ("Gate Range\nmode 2")
          }
          frame "l" {
            w648 = u16 1 items=["Auto", "Limited", "Fixed"] ("Gate Range\nmode 2")
          }
        }
      }
      frame "gaterange" {
        (unwired) u8 11 items=["10fA  ", "100fA  ", "1nA  ", "10nA", "100nA", "1uA", "10uA", "100uA", "1mA", "10mA", "100mA", "1A"] ("Gate Range 2")
        n180 = Delete From Array(array=w669, index=0 ("Index")) -> (deleted portion=w659:string)  [unwired: 1 in, 1 out]
        n181 = Scan Value(string=w659, format string="") -> (value=w657:dbl)  [unwired: 1 in, 1 out]
        n182 = Logarithm Base 10(1:w657) -> (0:w656:dbl)
        n183 = Round To Nearest(number=w656) -> (nearest integer value=w655:dbl)
        n184 = Add(x=w655, y=11.0) -> (x+y=w653:dbl)
        n185 = To Unsigned Byte Integer(number=w653) -> (unsigned 8bit integer=w652:u8)
      }
      frame "drainrange" {
        (unwired) u8 11 items=["10fA  ", "100fA  ", "1nA  ", "10nA", "100nA", "1uA", "10uA", "100uA", "1mA", "10mA", "100mA", "1A"] ("Gate Range 2")
        n186 = Delete From Array(array=w691, index=0 ("Index")) -> (deleted portion=w682:string)  [unwired: 1 in, 1 out]
        n187 = Scan Value(string=w682, format string="") -> (value=w680:dbl)  [unwired: 1 in, 1 out]
        n188 = Logarithm Base 10(1:w680) -> (0:w679:dbl)
        n189 = Round To Nearest(number=w679) -> (nearest integer value=w678:dbl)
        n190 = Add(x=w678, y=11.0) -> (x+y=w676:dbl)
        n191 = To Unsigned Byte Integer(number=w676) -> (unsigned 8bit integer=w675:u8)
      }
      frame "drainrangemode" {
        n192 = Delete From Array(array=w706, index=0 ("Index")) -> (deleted portion=w707:string)  [unwired: 1 in, 1 out]
        n193 = case shown="\"f\"" w707 {
          tunnel: [w709 w710 w711] -> w696
          frame "a", Default {
            w709 = u16 0 items=["Auto", "Limited", "Fixed"] ("Gate Range\nmode 2")
          }
          frame "f" {
            w710 = u16 2 items=["Auto", "Limited", "Fixed"] ("Gate Range\nmode 2")
          }
          frame "l" {
            w711 = u16 1 items=["Auto", "Limited", "Fixed"] ("Gate Range\nmode 2")
          }
        }
      }
      frame "Error", Default {
      }
      frame "logfile" {
        n194 = Number To Decimal String(number=w728) -> (decimal integer string=w763:string)  [unwired: 1 in]
        n195 = Concatenate Strings(w762, "logfile" ("Substring"), w763, w726, ".txt" ("Substring")) -> (w760:string)
        n196 = String To Path(string=w760) -> (path=w733:path)
        n197 = Unbundle(w759) -> ("integration time"=w758:u32, "Short/Long integration time"=w757:dbl, "hold time (sec)"=w756:dbl, "delay time (sec)"=w755:dbl, "Step Time (0 disables)"=w754:dbl, "sweep method"=w753:u16, "Pulse period"=w752:dbl, "Base voltage"=w751:dbl, "Pulse width"=w750:dbl)
        n198 = Build Array(w758, w757, w756, w755, w754, w753, w752, w751, w750, w744, w745, w746, w747, w748, w749) -> (w737:dbl[])
        n199 = Insert Into Array(array=dbl[][] [] ("Input Array"), new element=w737) -> (w736:dbl[][])  [unwired: 2 in]
        n200 = call <vilib>:"compatOverwrite.vi"("overwrite (F)"=TRUE) -> ("overwrite?"=w731:T7)
        n201 = Open/Create/Replace File(file path (use dialog)=w733, error in=w735, operation (0:open)=w731) -> (refnum out=w741:refnum<file>, error out=w740:errorcluster)  [unwired: 3 in, 1 out]
        n202 = call "4155C Write array to file.vi"("Byte Stream File Refnum"=w741, "Header"=string[] ["Int Time", "Short/Long Itime", "Hold time", "Delay time", "Step time", "Sweep method", "Pulse period", "Base Voltage", "Pulse width", "Drain compliance", "Gate compliance", "Gate range mode", "Gate range", "S/D range mode", "S/D range"], "Data Array"=w736, "error in (no error)"=w740) -> ("dup refnum"=w743:refnum<file>, "error out"=w742:errorcluster)  [unwired: 1 in]
        n203 = Close File(refnum=w743, error in=w742) -> (error out=w734:errorcluster)  [unwired: 1 out]
      }
      frame "sample" {
        n204 = Number To Decimal String(number=w768) -> (decimal integer string=w816:string)  [unwired: 1 in]
        n205 = Fract/Exp String To Number(string=w813) -> (number=w774:dbl[])  [unwired: 3 in, 1 out]
        n206 = Concatenate Strings(w791, "-sample-" ("Substring"), w816, w766, ".txt" ("Substring")) -> (w814:string)
        n207 = String To Path(string=w814) -> (path=w795:path)
        n208 = Index Array(array=w774, index=0 ("Index")) -> (element=w811:dbl)
        n209 = Index Array(array=w774, index=2 ("Index")) -> (element=w807:dbl)
        n210 = Index Array(array=w774, index=3 ("Index")) -> (element=w776:dbl)
        n211 = Index Array(array=w774, index=4 ("Index")) -> (element=w773:dbl)
        n212 = call "4155C Config Sampling Measurements.vi"("Sampling interval"=w773, "Sample time"=w776, "Display on/off"=TRUE, "Timings"=w782, "Num Points"=w807, "error in (no error)"=w818, "Drain Compliance"=w817, "Gate Compliance"=w792, "VISA session"=w819) -> ("error out"=w820:errorcluster, "dup VISA resource name"=w821:refnum<visa-resource-name>)  [unwired: 1 in]
        n213 = Index Array(array=w774, index=1 ("Index")) -> (element=w808:dbl)
        n214 = call "4155C Take Sample.vi"("Emergency Stop"=w788, "error in (no error)"=w820, "Vd"=w808, "Vg"=w811, "VISA resource name in"=w821) -> ("error out"=w786:errorcluster, "Id"=w823:dbl[], "Ig"=w797:dbl[], "VISA Resource Name out"=w784:refnum<visa-resource-name>, "Is"=w822:dbl[], "Time"=w801:dbl[])  [unwired: 1 in]
        n215 = Insert Into Array(array=dbl[][] [] ("Input Array"), new element=w801) -> (w800:dbl[][])  [unwired: 2 in]
        n216 = Insert Into Array(array=w800, new element=w797) -> (w799:dbl[][])  [unwired: 2 in]
        n217 = Insert Into Array(array=w799, new element=w823) -> (w798:dbl[][])  [unwired: 2 in]
        n218 = VISA Write(VISA resource name=w784, write buffer=":DISP ON" ("write buffer (\"\")"), error in (no error)=w786) -> (VISA resource name out=w783:refnum<visa-resource-name>, error out=w785:errorcluster)  [unwired: 1 out]
        n219 = Insert Into Array(array=w798, new element=w822) -> (w790:dbl[][])  [unwired: 2 in]
        n220 = Transpose 2D Array(2D array=w790) -> (transposed array=w789:dbl[][])
        n221 = call <vilib>:"compatOverwrite.vi"("overwrite (F)"=TRUE) -> ("overwrite?"=w771:T7)
        n222 = Open/Create/Replace File(file path (use dialog)=w795, error in=w785, operation (0:open)=w771) -> (refnum out=w804:refnum<file>, error out=w803:errorcluster)  [unwired: 3 in, 1 out]
        n223 = call "4155C Write array to file.vi"("Byte Stream File Refnum"=w804, "Header"=string[] ["Time /s", "Ig /A", "Id /A", "Is /A"], "Data Array"=w789, "error in (no error)"=w803) -> ("dup refnum"=w806:refnum<file>, "error out"=w805:errorcluster)  [unwired: 1 in]
        n224 = Close File(refnum=w806, error in=w805) -> (error out=w793:errorcluster)  [unwired: 1 out]
      }
      frame "samplei" {
        n225 = Number To Decimal String(number=w826) -> (decimal integer string=w878:string)  [unwired: 1 in]
        n226 = Fract/Exp String To Number(string=w875) -> (number=w842:dbl[])  [unwired: 3 in, 1 out]
        n227 = Concatenate Strings(w857, "-samplei-" ("Substring"), w878, w825, ".txt" ("Substring")) -> (w876:string)
        n228 = String To Path(string=w876) -> (path=w860:path)
        n229 = Index Array(array=w842, index=4 ("Index")) -> (element=w836:dbl)
        n230 = Index Array(array=w842, index=3 ("Index")) -> (element=w837:dbl)
        n231 = Index Array(array=w842, index=1 ("Index")) -> (element=w839:dbl)
        n232 = Index Array(array=w842, index=0 ("Index")) -> (element=w840:dbl)
        n233 = Index Array(array=w842, index=2 ("Index")) -> (element=w838:dbl)
        n234 = call "4155C Config SamplingI Measurements.vi"("Sample time"=w838, "Display on/off"=TRUE, "Timings"=w849, "Num Points"=w839, "error in (no error)"=w880, "Sampling interval"=w837, "VISA session"=w881) -> ("error out"=w882:errorcluster, "dup VISA resource name"=w883:refnum<visa-resource-name>)  [unwired: 3 in]
        n235 = call "4155C Take SampleI.vi"("Emergency Stop"=w854, "error in (no error)"=w882, "Idg 2"=w840, "Vdg compliance 2"=w836, "VISA resource name in"=w883) -> ("error out"=w852:errorcluster, "Idg"=w885:dbl[], "Vdg"=w862:dbl[], "VISA Resource Name out"=w850:refnum<visa-resource-name>, "Is"=w884:dbl[], "Time"=w866:dbl[])  [unwired: 1 in]
        n236 = Insert Into Array(array=dbl[][] [] ("Input Array"), new element=w866) -> (w865:dbl[][])  [unwired: 2 in]
        n237 = Insert Into Array(array=w865, new element=w862) -> (w864:dbl[][])  [unwired: 2 in]
        n238 = Insert Into Array(array=w864, new element=w885) -> (w863:dbl[][])  [unwired: 2 in]
        n239 = VISA Write(VISA resource name=w850, write buffer=":DISP ON" ("write buffer (\"\")"), error in (no error)=w852) -> (VISA resource name out=w835:refnum<visa-resource-name>, error out=w851:errorcluster)  [unwired: 1 out]
        n240 = Insert Into Array(array=w863, new element=w884) -> (w856:dbl[][])  [unwired: 2 in]
        n241 = Transpose 2D Array(2D array=w856) -> (transposed array=w855:dbl[][])
        n242 = call <vilib>:"compatOverwrite.vi"("overwrite (F)"=TRUE) -> ("overwrite?"=w830:T7)
        n243 = Open/Create/Replace File(file path (use dialog)=w860, error in=w851, operation (0:open)=w830) -> (refnum out=w869:refnum<file>, error out=w868:errorcluster)  [unwired: 3 in, 1 out]
        n244 = call "4155C Write array to file.vi"("Byte Stream File Refnum"=w869, "Header"=string[] ["Time /s", "Vdg /V", "Idg /A", "Is /A"], "Data Array"=w855, "error in (no error)"=w868) -> ("dup refnum"=w871:refnum<file>, "error out"=w870:errorcluster)  [unwired: 1 in]
        n245 = Close File(refnum=w871, error in=w870) -> (error out=w833:errorcluster)  [unwired: 1 out]
        n246 = VISA Write(VISA resource name=w835, write buffer=";:PAGE:SCON:STAN OFF;:PAGE:CHAN:VSU2:DIS;" ("write buffer (\"\")"), error in (no error)=w833) -> (VISA resource name out=w831:refnum<visa-resource-name>, error out=w832:errorcluster)  [unwired: 1 out]
      }
      frame "#" {
        n247 = VISA Write(VISA resource name=w893, write buffer=":DISP ON" ("write buffer (\"\")"), error in (no error)=w892) -> (VISA resource name out=w891:refnum<visa-resource-name>, error out=w890:errorcluster)  [unwired: 1 out]
      }
      frame "stressV" {
        n248 = Number To Decimal String(number=w904) -> (decimal integer string=w945:string)  [unwired: 1 in]
        n249 = Fract/Exp String To Number(string=w942) -> (number=w915:dbl[])  [unwired: 3 in, 1 out]
        n250 = Concatenate Strings(w929, "-stressV-" ("Substring"), w945, w903, ".txt" ("Substring")) -> (w943:string)
        n251 = String To Path(string=w943) -> (path=w933:path)
        n252 = Index Array(array=w915, index=3 ("Index")) -> (element=w912:dbl)
        n253 = Index Array(array=w915, index=1 ("Index")) -> (element=w910:dbl)
        n254 = Index Array(array=w915, index=0 ("Index")) -> (element=w909:dbl)
        n255 = Index Array(array=w915, index=4 ("Index")) -> (element=w914:dbl)
        n256 = Index Array(array=w915, index=2 ("Index")) -> (element=w911:dbl)
        n257 = call "4155C Config V Stress.vi"("VISA session"=w948, "ID compliance"=w912, "VD"=w910, "VG"=w909, "IG compliance"=w911, "error in (no error)"=w947, "Display on/off"=TRUE) -> ("dup VISA resource name"=w950:refnum<visa-resource-name>, "error out"=w949:errorcluster)
        n258 = call "4155C Apply Stress.vi"("error in (no error)"=w949, "Duration"=w914, "Emergency Stop"=w928, "VISA resource name in"=w950) -> ("error out"=w926:errorcluster, "VISA Resource Name out"=w924:refnum<visa-resource-name>)
        n259 = VISA Write(VISA resource name=w924, write buffer=":DISP ON" ("write buffer (\"\")"), error in (no error)=w926) -> (VISA resource name out=w923:refnum<visa-resource-name>, error out=w925:errorcluster)  [unwired: 1 out]
        n260 = call <vilib>:"compatOverwrite.vi"("overwrite (F)"=TRUE) -> ("overwrite?"=w908:T7)
        n261 = Open/Create/Replace File(file path (use dialog)=w933, error in=w925, operation (0:open)=w908) -> (refnum out=w936:refnum<file>, error out=w935:errorcluster)  [unwired: 3 in, 1 out]
        n262 = call "4155C Write array to file.vi"("Byte Stream File Refnum"=w936, "Header"=string[] ["V stress completed successfully", ""], "error in (no error)"=w935) -> ("dup refnum"=w938:refnum<file>, "error out"=w937:errorcluster)  [unwired: 2 in]
        n263 = Close File(refnum=w938, error in=w937) -> (error out=w931:errorcluster)  [unwired: 1 out]
      }
      frame "stressI" {
        n264 = Number To Decimal String(number=w953) -> (decimal integer string=w990:string)  [unwired: 1 in]
        n265 = Fract/Exp String To Number(string=w987) -> (number=w962:dbl[])  [unwired: 3 in, 1 out]
        n266 = Concatenate Strings(w974, "-stressI-" ("Substring"), w990, w952, ".txt" ("Substring")) -> (w988:string)
        n267 = String To Path(string=w988) -> (path=w978:path)
        n268 = Index Array(array=w962, index=1 ("Index")) -> (element=w958:dbl)
        n269 = Index Array(array=w962, index=0 ("Index")) -> (element=w959:dbl)
        n270 = call "4155C Config I Stress.vi"("VISA session"=w993, "IDG"=w959, "VDG compliance"=w958, "error in (no error)"=w992, "Display on/off"=TRUE) -> ("dup VISA resource name"=w995:refnum<visa-resource-name>, "error out"=w994:errorcluster)
        n271 = Index Array(array=w962, index=2 ("Index")) -> (element=w960:dbl)
        n272 = call "4155C Apply Stress.vi"("error in (no error)"=w994, "Duration"=w960, "Emergency Stop"=w973, "VISA resource name in"=w995) -> ("error out"=w971:errorcluster, "VISA Resource Name out"=w969:refnum<visa-resource-name>)
        n273 = VISA Write(VISA resource name=w969, write buffer=":DISP ON" ("write buffer (\"\")"), error in (no error)=w971) -> (VISA resource name out=w968:refnum<visa-resource-name>, error out=w970:errorcluster)  [unwired: 1 out]
        n274 = call <vilib>:"compatOverwrite.vi"("overwrite (F)"=TRUE) -> ("overwrite?"=w957:T7)
        n275 = Open/Create/Replace File(file path (use dialog)=w978, error in=w970, operation (0:open)=w957) -> (refnum out=w981:refnum<file>, error out=w980:errorcluster)  [unwired: 3 in, 1 out]
        n276 = call "4155C Write array to file.vi"("Byte Stream File Refnum"=w981, "Header"=string[] ["I stress completed successfully", ""], "error in (no error)"=w980) -> ("dup refnum"=w983:refnum<file>, "error out"=w982:errorcluster)  [unwired: 2 in]
        n277 = Close File(refnum=w983, error in=w982) -> (error out=w976:errorcluster)  [unwired: 1 out]
      }
      frame "vsu2pulse" {
        n278 = Number To Decimal String(number=w998) -> (decimal integer string=w1033:string)  [unwired: 1 in]
        n279 = Fract/Exp String To Number(string=w1030) -> (number=w1006:dbl[])  [unwired: 3 in, 1 out]
        n280 = Concatenate Strings(w1018, "-vsu2-" ("Substring"), w1033, w997, ".txt" ("Substring")) -> (w1031:string)
        n281 = String To Path(string=w1031) -> (path=w1022:path)
        n282 = Index Array(array=w1006, index=1 ("Index")) -> (element=w1005:dbl)
        n283 = Index Array(array=w1006, index=0 ("Index")) -> (element=w1003:dbl)
        n284 = call "4155C Config VSU2 Stress.vi"("error in (no error)"=w1035, "VSU2"=w1003, "Display on/off"=TRUE, "VISA session"=w1036) -> ("error out"=w1037:errorcluster, "dup VISA resource name"=w1038:refnum<visa-resource-name>)
        n285 = call "4155C Apply Stress.vi"("error in (no error)"=w1037, "Duration"=w1005, "Emergency Stop"=w1017, "VISA resource name in"=w1038) -> ("error out"=w1015:errorcluster, "VISA Resource Name out"=w1013:refnum<visa-resource-name>)
        n286 = VISA Write(VISA resource name=w1013, write buffer=":DISP ON" ("write buffer (\"\")"), error in (no error)=w1015) -> (VISA resource name out=w1012:refnum<visa-resource-name>, error out=w1014:errorcluster)  [unwired: 1 out]
        n287 = call <vilib>:"compatOverwrite.vi"("overwrite (F)"=TRUE) -> ("overwrite?"=w1002:T7)
        n288 = Open/Create/Replace File(file path (use dialog)=w1022, error in=w1014, operation (0:open)=w1002) -> (refnum out=w1025:refnum<file>, error out=w1024:errorcluster)  [unwired: 3 in, 1 out]
        n289 = call "4155C Write array to file.vi"("Byte Stream File Refnum"=w1025, "Header"=string[] ["VSU2 pulse completed successfully", ""], "error in (no error)"=w1024) -> ("dup refnum"=w1027:refnum<file>, "error out"=w1026:errorcluster)  [unwired: 2 in]
        n290 = Close File(refnum=w1027, error in=w1026) -> (error out=w1020:errorcluster)  [unwired: 1 out]
      }
      frame "sample-fpp" {
        w1052 = string[] ["Time /s", "Id VgVd /A", "Ig VgVd /A", "Vp1 VgVd /V", "Vp2 VgVd /V"] ("Header")
        w1056 = "%d" ("format string")
        n291 = Number To Decimal String(number=w1041) -> (decimal integer string=w1104:string)  [unwired: 1 in]
        n292 = Fract/Exp String To Number(string=w1101) -> (number=w1089:dbl[])  [unwired: 3 in, 1 out]
        n293 = Concatenate Strings(w1095, "-samplefpp-" ("Substring"), w1104, w1040, ".txt" ("Substring")) -> (w1102:string)
        n294 = String To Path(string=w1102) -> (path=w1064:path)
        n295 = Index Array(array=w1089, index=0 ("Index")) -> (element=w1050:dbl)
        n296 = Index Array(array=w1089, index=1 ("Index")) -> (element=w1049:dbl)
        n297 = Index Array(array=w1089, index=2 ("Index")) -> (element=w1097:dbl)
        n298 = Index Array(array=w1089, index=3 ("Index")) -> (element=w1087:dbl)
        n299 = call "4155C Config Sampling Measurements FPP.vi"("VISA session"=w1107, "Num Points"=w1097, "Vg"=w1050, "Display on/off"=TRUE, "Gate Compliance"=w1096, "Drain Compliance"=w1105, "Standby"="Standby", "error in (no error)"=w1106, "Timings"=w1094, "Vd"=w1049, "Sample time"=w1087) -> ("dup VISA resource name"=w1066:refnum<visa-resource-name>, "error out"=w1065:errorcluster)  [unwired: 3 in]
        n300 = Number To Decimal String(number=w1050) -> (decimal integer string=w1076:string)  [unwired: 1 in]
        n301 = call "4155C Take Sample FPP.vi"("VISA resource name in"=w1066, "error in (no error)"=w1065, "Emergency Stop"=w1067) -> ("Time"=w1071:dbl[], "Vp1"=w1081:dbl[], "VISA Resource Name out"=w1047:refnum<visa-resource-name>, "Ig"=w1069:dbl[], "Id"=w1070:dbl[], "Vp2"=w1079:dbl[], "error out"=w1068:errorcluster)  [unwired: 10 in]
        n302 = Insert Into Array(array=dbl[][] [] ("Input Array"), new element=w1071) -> (w1085:dbl[][])  [unwired: 2 in]
        n303 = Number To Decimal String(number=w1049) -> (decimal integer string=w1074:string)  [unwired: 1 in]
        n304 = Insert Into Array(array=w1085, new element=w1070) -> (w1084:dbl[][])  [unwired: 2 in]
        n305 = Concatenate Strings("(Vg = " ("Substring"), w1076, "V, Vd = " ("Substring"), w1074, "V)" ("Substring")) -> (w1072:string)
        n306 = Insert Into Array(array=w1084, new element=w1069) -> (w1083:dbl[][])  [unwired: 2 in]
        n307 = Insert Into Array(array=w1083, new element=w1081) -> (w1080:dbl[][])  [unwired: 2 in]
        n308 = Insert Into Array(array=w1080, new element=w1079) -> (w1048:dbl[][])  [unwired: 2 in]
        n309 = call <vilib>:"compatOverwrite.vi"("overwrite (F)"=TRUE) -> ("overwrite?"=w1045:T7)
        n310 = Open/Create/Replace File(file path (use dialog)=w1064, error in=w1068, operation (0:open)=w1045) -> (refnum out=w1061:refnum<file>, error out=w1062:errorcluster)  [unwired: 3 in, 1 out]
        n311 = Array To Spreadsheet String(array=w1052, 3:w1056) -> (spreadsheet string=w1058:string)  [unwired: 1 in]
        n312 = Transpose 2D Array(2D array=w1048) -> (transposed array=w1078:dbl[][])
        n313 = Search and Replace String(replace all?=TRUE ("replace all? (F)"), input string=w1058, search string="VgVd", replace string=w1072) -> (result string=w1054:string)  [unwired: 4 in, 3 out]
        n314 = Spreadsheet String To Array(format string=w1056, spreadsheet string=w1054, array type (2D Dbl)=w1052) -> (array=w1053:string[])  [unwired: 1 in]
        n315 = call "4155C Write array to file.vi"("Byte Stream File Refnum"=w1061, "Header"=w1053, "Data Array"=w1078, "error in (no error)"=w1062) -> ("dup refnum"=w1059:refnum<file>, "error out"=w1060:errorcluster)  [unwired: 1 in]
        n316 = Close File(refnum=w1059, error in=w1060) -> (error out=w1046:errorcluster)  [unwired: 1 out]
      }
      frame "resample-fpp" {
        w1123 = string[] ["Time /s", "Id VgVd /A", "Ig VgVd /A", "Vp1 VgVd /V", "Vp2 VgVd /V"] ("Header")
        w1127 = "%d" ("format string")
        n317 = Number To Decimal String(number=w1109) -> (decimal integer string=w1167:string)  [unwired: 1 in]
        n318 = Fract/Exp String To Number(string=w1164) -> (number=w1116:dbl[])  [unwired: 3 in, 1 out]
        n319 = Concatenate Strings(w1160, "-resamplefpp-" ("Substring"), w1167, w1110, ".txt" ("Substring")) -> (w1165:string)
        n320 = String To Path(string=w1165) -> (path=w1135:path)
        n321 = Index Array(array=w1116, index=0 ("Index")) -> (element=w1122:dbl)
        n322 = Index Array(array=w1116, index=1 ("Index")) -> (element=w1121:dbl)
        n323 = Number To Decimal String(number=w1122) -> (decimal integer string=w1145:string)  [unwired: 1 in]
        n324 = call "4155C Take Sample FPP.vi"("VISA resource name in"=w1118, "error in (no error)"=w1117, "Emergency Stop"=w1136) -> ("Time"=w1140:dbl[], "Vp1"=w1150:dbl[], "VISA Resource Name out"=w1120:refnum<visa-resource-name>, "Ig"=w1138:dbl[], "Id"=w1139:dbl[], "Vp2"=w1148:dbl[], "error out"=w1137:errorcluster)  [unwired: 10 in]
        n325 = Insert Into Array(array=dbl[][] [] ("Input Array"), new element=w1140) -> (w1154:dbl[][])  [unwired: 2 in]
        n326 = Number To Decimal String(number=w1121) -> (decimal integer string=w1143:string)  [unwired: 1 in]
        n327 = Insert Into Array(array=w1154, new element=w1139) -> (w1153:dbl[][])  [unwired: 2 in]
        n328 = Concatenate Strings("(Vg = " ("Substring"), w1145, "V, Vd = " ("Substring"), w1143, "V)" ("Substring")) -> (w1141:string)
        n329 = Insert Into Array(array=w1153, new element=w1138) -> (w1152:dbl[][])  [unwired: 2 in]
        n330 = Insert Into Array(array=w1152, new element=w1150) -> (w1149:dbl[][])  [unwired: 2 in]
        n331 = Insert Into Array(array=w1149, new element=w1148) -> (w1115:dbl[][])  [unwired: 2 in]
        n332 = call <vilib>:"compatOverwrite.vi"("overwrite (F)"=TRUE) -> ("overwrite?"=w1114:T7)
        n333 = Open/Create/Replace File(file path (use dialog)=w1135, error in=w1137, operation (0:open)=w1114) -> (refnum out=w1132:refnum<file>, error out=w1133:errorcluster)  [unwired: 3 in, 1 out]
        n334 = Array To Spreadsheet String(array=w1123, 3:w1127) -> (spreadsheet string=w1129:string)  [unwired: 1 in]
        n335 = Transpose 2D Array(2D array=w1115) -> (transposed array=w1147:dbl[][])
        n336 = Search and Replace String(replace all?=TRUE ("replace all? (F)"), input string=w1129, search string="VgVd", replace string=w1141) -> (result string=w1125:string)  [unwired: 4 in, 3 out]
        n337 = Spreadsheet String To Array(format string=w1127, spreadsheet string=w1125, array type (2D Dbl)=w1123) -> (array=w1124:string[])  [unwired: 1 in]
        n338 = call "4155C Write array to file.vi"("Byte Stream File Refnum"=w1132, "Header"=w1124, "Data Array"=w1147, "error in (no error)"=w1133) -> ("dup refnum"=w1130:refnum<file>, "error out"=w1131:errorcluster)  [unwired: 1 in]
        n339 = Close File(refnum=w1130, error in=w1131) -> (error out=w1119:errorcluster)  [unwired: 1 out]
      }
      frame "serial" {
        n340 = Index Array(array=w1172, index=0 ("Index")) -> (element=w1171:string)
        n341 = call "Serial write and read v0.4.vi"("Termination char\n(0xA = '\\n' = LF)\n(0xD = '\\r' = CR)"="Termination char\n(0xA = '\\n' = LF)\n(0xD = '\\r' = CR)", "Enable Termination\nChar (T)"="Enable Termination\nChar (T)", "parity"="parity", "stop bits"="stop bits", "string to write"=w1171, "flow control"="flow control", "byte count"="byte count", "Serial Settings:Serial End Mode for Reads"="Serial End Mode for Reads", "Timeout (ms)"="Timeout (ms)", "error in (no error)"=w1177, "VISA resource name"="VISA resource name", "baud rate"="baud rate", "data bits"="data bits") -> ("read string"=→"Serial port output":string, "error out"=w1176:errorcluster)  [unwired: 1 in]
      }
    }
    n342 = Build Array("Time /s" ("element"), "Id max /A" ("VAR2 Name"), "Id min /A" ("VAR2 Name")) -> (w68:string[])
    n343 = Build Array(w63, w62, w54) -> (w61:dbl[][])
    n344 = Transpose 2D Array(2D array=w61) -> (transposed array=w60:dbl[][])
    n345 = Concatenate Strings(w59, "-Ion-Ioff", ".txt" ("Suffix")) -> (w76:string)
    n346 = Array To Spreadsheet String(array=w68, 3:"" ("format string")) -> (spreadsheet string=w67:string)  [unwired: 1 in]
    n347 = Array To Spreadsheet String(array=w60, 3:"%e" ("format string")) -> (spreadsheet string=w66:string)  [unwired: 1 in]
    n348 = String To Path(string=w76) -> (path=w75:path)
    n349 = Build Array(w67, w66) -> (w65:string[])
    n350 = Write to Text File(file (use dialog)=w75, text=w65, error in=w57) -> (refnum out=w77:refnum<file>, error out=w64:errorcluster)  [unwired: 1 in, 1 out]
    n351 = Close File(refnum=w77, error in=w64) -> (error out=w56:errorcluster)  [unwired: 1 out]
    "Line running" <- w87
    "Total lines" <- w86
  }
  "error out" <- w7
